vi "Text control 2 v2.7.vi"() -> ()   [LabVIEW 2016]
panel:
  out "Total lines":i32
  out "Line running":i32
  in  "byte count":u32=64
  in  "Serial Settings:Serial End Mode for Reads":u16(ring)=2 items=["None", "LastBit", "TermChar"]
  in  "Timeout (ms)":u32=10000
  in  "Enable Termination\nChar (T)":bool=TRUE
  in  "Termination char\n(0xA = '\\n' = LF)\n(0xD = '\\r' = CR)":u8=13 format="%.0x"
  in  "flow control":u16(ring) items=["None"=0, "XON/XOFF"=1, "RTS/CTS"=2, "DTR/DSR"=4]
  in  "stop bits":u16(ring)=10 items=["1.0"=10, "1.5"=15, "2.0"=20]
  in  "parity":u16(ring) items=["None", "Odd", "Even", "Mark", "Space"]
  in  "data bits":u16=8 min=5 max=8 step=1
  in  "VISA resource name":refnum<visa-resource-name>="COM6"
  in  "baud rate":u32=9600
  out "Serial port output":string
  out "error out":errorcluster
  in  "Units":bool
  out "Elapsed Time":dbl caption="Elapsed Time (s)"
  out "Id max vs time":cluster{"Y data in":dbl[], "X data in":dbl[]}[](graph)
  out "Ig":dbl format="%.2e"
  out "Id":dbl format="%.2e"
  out "Is":dbl format="%.2e"
  out "I vs Vg":cluster{"Y data in":dbl[], "X data in":dbl[]}[](graph)
  in  "Panel Controls 2":T1={"Emergency Stop"=refnum, "TransGraph Max"=1e-05, "Text/Graph (text=false)"=TRUE, "TransGraph Min"=1e-11} {"TransGraph Min" format="%.2e"; "TransGraph Max" format="%.2e"}
  out "Command running:":string="#output s 0 0 0 -0.008 0.008 0.002"
  in  "Standby":T2
  in  "Full Reset":bool
  in  "SMU4":cluster{"on/off":bool, "Voltage":dbl} {"Voltage" min=-100.0 max=100.0 format="%.2f"}
  in  "Source/Drain Range":u8(slide)=6 max=11 scale=0.0..11.0
  in  "Source/Drain\nRange mode":u16(ring) items=["Auto", "Limited", "Fixed"]
  in  "Gate Range":u8(slide)=6 max=11 scale=0.0..11.0
  in  "Gate Range\nmode":u16(ring) items=["Auto", "Limited", "Fixed"]
  in  "Gate":T3={"Gate Start"=0.0, "Gate Stop"=2.0, "Gate Step (linear only)"=1.0, "Gate Compliance"=0.0001, "Gate PComp"=0.0, "Range mode"=0, "Range"=6} {"Range" max=11 scale=0.0..11.0; "Range mode" items=["Auto", "Limited", "Fixed"]; "Gate PComp" format="%^.2e"; "Gate Compliance" format="%^.2e"; "Gate Step (linear only)" format="%^.4e"; "Gate Stop" format="%^.4e"; "Gate Start" format="%^.4e"}
  in  "Drain 2":T4={"Drain Start"=0.0, "Drain Stop"=2.0, "Drain Compliance"=0.0001, "Drain Step"=1.0, "Drain PComp"=0.0, "Range mode"=0, "Range"=6} {"Range" max=11 scale=0.0..11.0; "Range mode" items=["Auto", "Limited", "Fixed"]; "Drain PComp" format="%^.2e"; "Drain Step" format="%^.4e"; "Drain Compliance" format="%^.2e"; "Drain Stop" format="%^.4e"; "Drain Start" format="%^.4e"}
  in  "Timings 2":T5={"integration time"=0, "Short/Long integration time"=0.00064, "hold time (sec)"=0.0, "delay time (sec)"=0.0, "Step Time (0 disables)"=0.0, "sweep method"=0, "Pulse period"=0.005, "Base voltage"=0.0, "Pulse width"=0.0005} {"Pulse width" min=0.0005 max=0.1 step=0.0001 format="%.4f"; "Base voltage" format="%^.4e"; "Pulse period" min=0.005 max=1.0 step=0.0001 format="%.4f"; "sweep method" items=["Continuous", "Pulsed"]; "Step Time (0 disables)" format="%.2f"; "delay time (sec)" format="%.4f"; "hold time (sec)" format="%.4f"; "Short/Long integration time" format="%^.0e"; "integration time" scale=0.0..2.0}
  in  "Panel Controls":T6={"Emergency Stop"=refnum, "TransGraph Max"=1e-05, "Text/Graph (text=false)"=TRUE} {"TransGraph Max" format="%.2e"}
  in  "Interrupt run":bool
  in  "Drain: Compliance":dbl=0.001 format="%.8f"
  in  "Gate: Compliance":dbl=0.001 format="%.8f"
  out "Path":path=path "C:/users/rlp38/09Apr2009LTtesting/test2.txt"
  in  "hold time /s":dbl format="%.2f"
  in  "delay time /s":dbl format="%.2f"
  in  "integration time":u32(slide) max=2 step=1 scale=0.0..2.0
  in  "Integration time (short)":dbl=0.0019 min=8e-05 max=0.0019 step=8e-05 format="%^.0e"
  in  "Integration time (long)":dbl=0.32 min=0.04 max=2.0 step=0.02 format="%.2f"
  in  "Step delay /s":dbl format="%.2f"
  in  "Program":string="#pulsedstressV d 0.03 20 0 0.5 0.0827 5\n#\n#itime s\n#gaterangemode l\n#drainrangemode l\n#pulsed on 0.05 0 0.02\n#transfer d 1 -1 -0.1 -1 -1 0\n#wait-min 1\n#transfer d 1 -1 -0.1 -1 -1 0\n#output d 0 -1 -0.5 0 -1 -0.1\n#transfer d -10 40 1 5 40 35\n#transfer d -10 40 1 5 40 35\n#output d 0 40 20 0 40 1\n#\n#\n#sample 1 0.008 221 6 0.003\n#samplei 400e-6 200 6 0.002 0.1\n#vsu2pulse -10 4\n#\n#stressV 0.016 0.03 2e-4 0.1e-3 11\n#stressI 220e-7 0.08 15\n#transfer s -1 1 0.5 -0.005 0.005 0.005\n#output s 0 0 0 -0.008 0.008 0.002\n"
  # "Serial port settings"
  # "Time"
  # "Sec"
  # "Min"
  # "100 samples is approx 13s with medium integration"
  # "Syntax:\nitime [s|m|l]\ngaterangemode [a|l|f]\ndrainrangemode [a|l|f]\npulsed [on|off] PulsePeriod(sec) PulseBaseVoltage PulseONWidth(sec)\nstandby [on l off]\nwait NumMilliseconds\nwait-min NumMinutes\n# texthere = comment\ntransfer [s|d] VgStart VgStop VgStep VdStart VdStop VdStep\noutput [s|d] VgStart VgStop VgStep VdStart VdStop VdStep\nsample Vg Vd NumSamples Time(s) SampleInterval(s)\nsamplei Idg NumSamples Time(s) SampleInterval(s) VDGcompliance\n# if in doubt use SampleInterval(s) = 0.004\nstressV VG VD IGcompliance IDcompliance Duration(sec)\nstressI IDG VDGcompliance Duration(sec)\nvsu2pulse Bias Duration(s)\npulsedstressV [s|d] VEstop VgON VgOFF Period(s) PulseONwidth(s) Vd\nsample-fpp Vg Vd NumSamples Time\nresample-fpp Vg Vd\ntransfer-fpp [s|d] VgStart VgStop VgStep VdStart VdStop VdStep\noutput-fpp [s|d] VgStart VgStop VgStep VdStart VdStop VdStep\nserial SerialPortCommand"
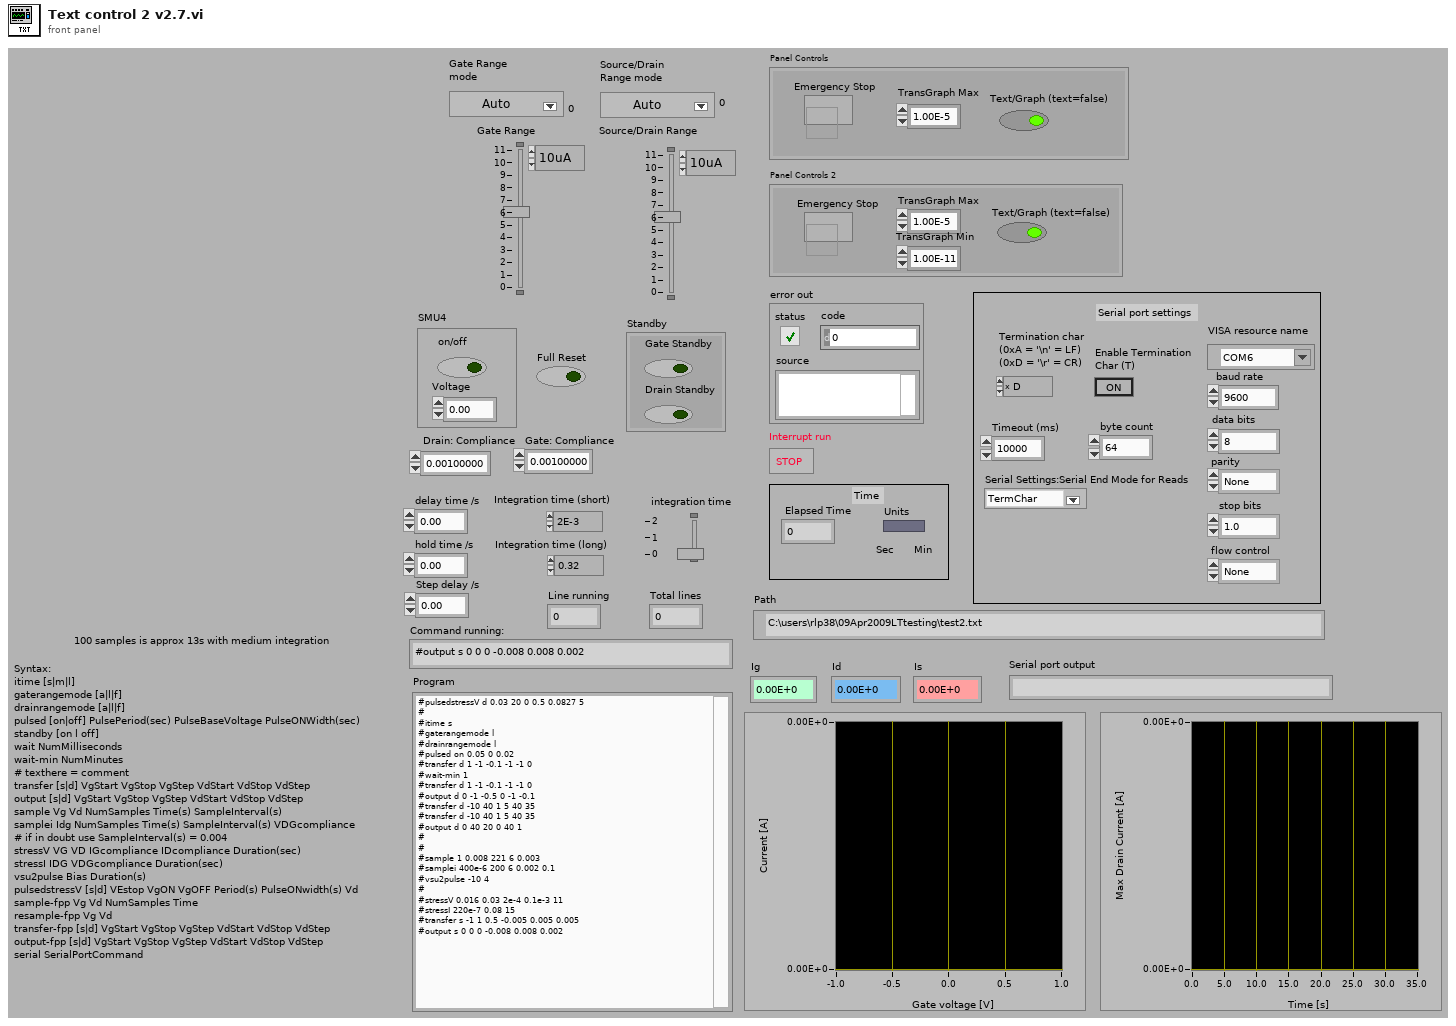
[diagram p1: front panel]
types:
  T1 = cluster{"Emergency Stop":refnum<vi>, "TransGraph Max":dbl, "Text/Graph (text=false)":bool, "TransGraph Min":dbl}
  T2 = cluster{"Gate Standby":bool, "Drain Standby":bool}
  T3 = cluster{"Gate Start":dbl, "Gate Stop":dbl, "Gate Step (linear only)":dbl, "Gate Compliance":dbl, "Gate PComp":dbl, "Range mode":u16, "Range":u8}
  T4 = cluster{"Drain Start":dbl, "Drain Stop":dbl, "Drain Compliance":dbl, "Drain Step":dbl, "Drain PComp":dbl, "Range mode":u16, "Range":u8}
  T5 = cluster{"integration time":u32, "Short/Long integration time":dbl, "hold time (sec)":dbl, "delay time (sec)":dbl, "Step Time (0 disables)":dbl, "sweep method":u16, "Pulse period":dbl, "Base voltage":dbl, "Pulse width":dbl}
  T6 = cluster{"Emergency Stop":refnum<vi>, "TransGraph Max":dbl, "Text/Graph (text=false)":bool}
  T7 = enum16{"open", "replace", "create", "open or create", "replace or create", "replace or create with confirmation"}
  T8 = cluster{"V2 Start":dbl, "V2 Step":dbl, "Number of points":i32}
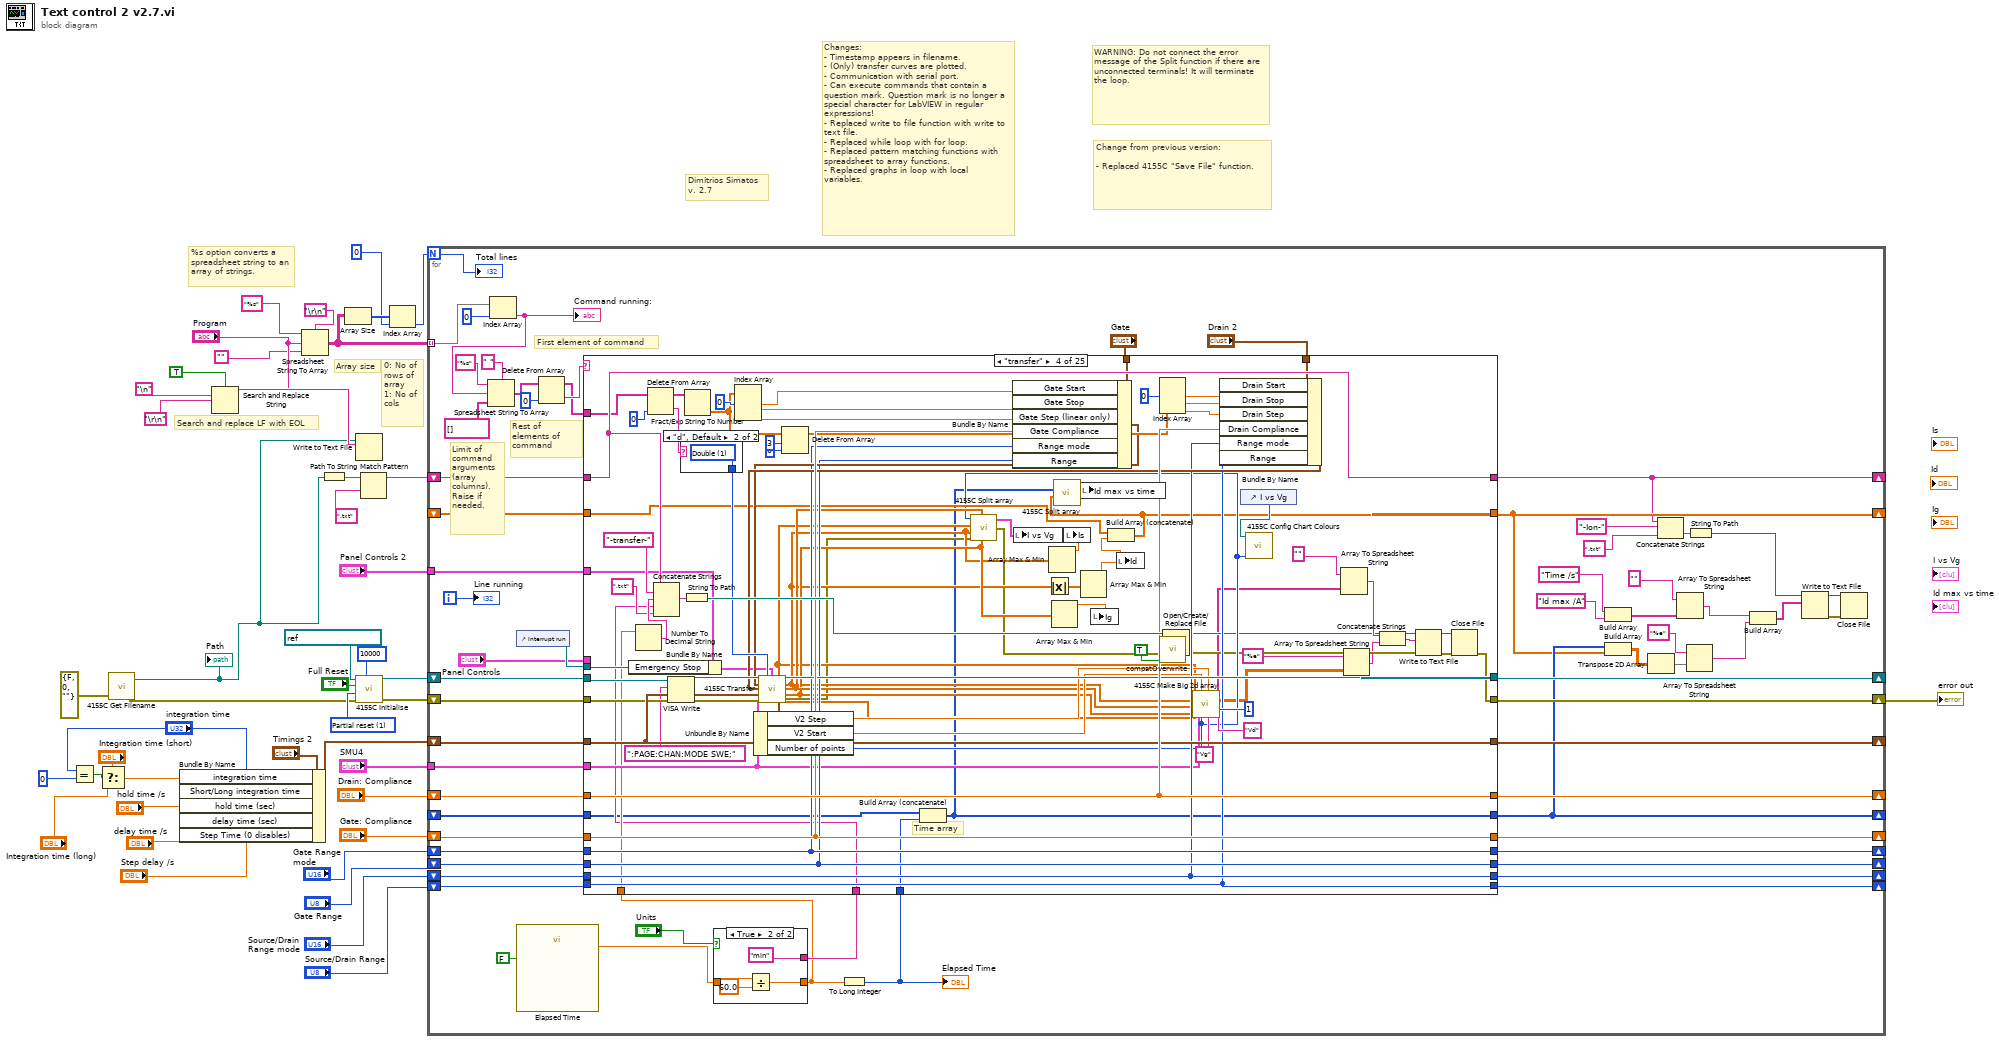
[diagram p0: block diagram]
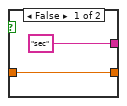
[diagram p2: hidden frame]
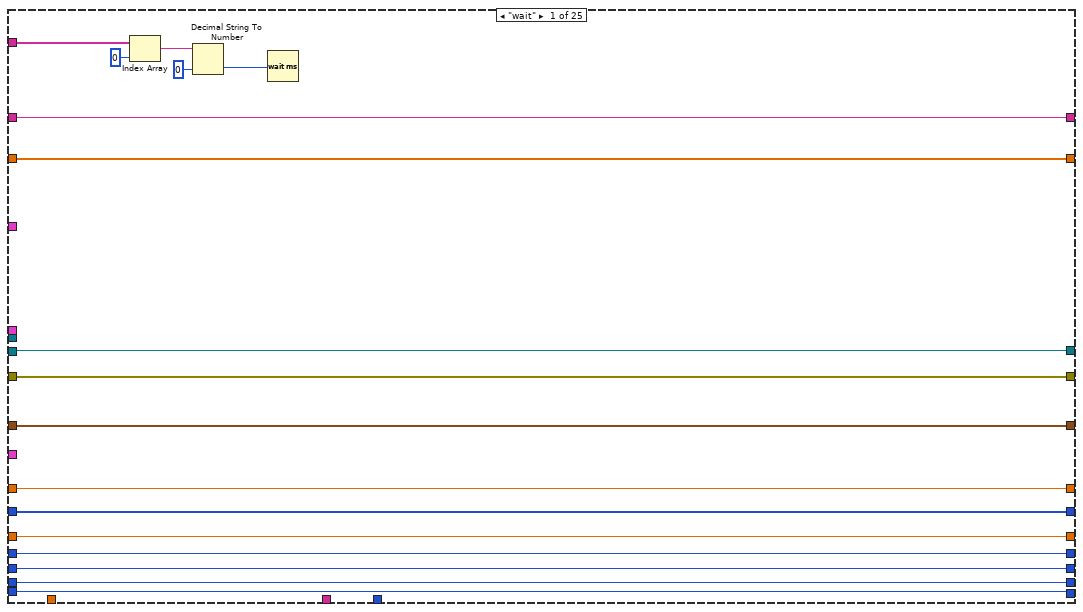
[diagram p3: hidden frame]
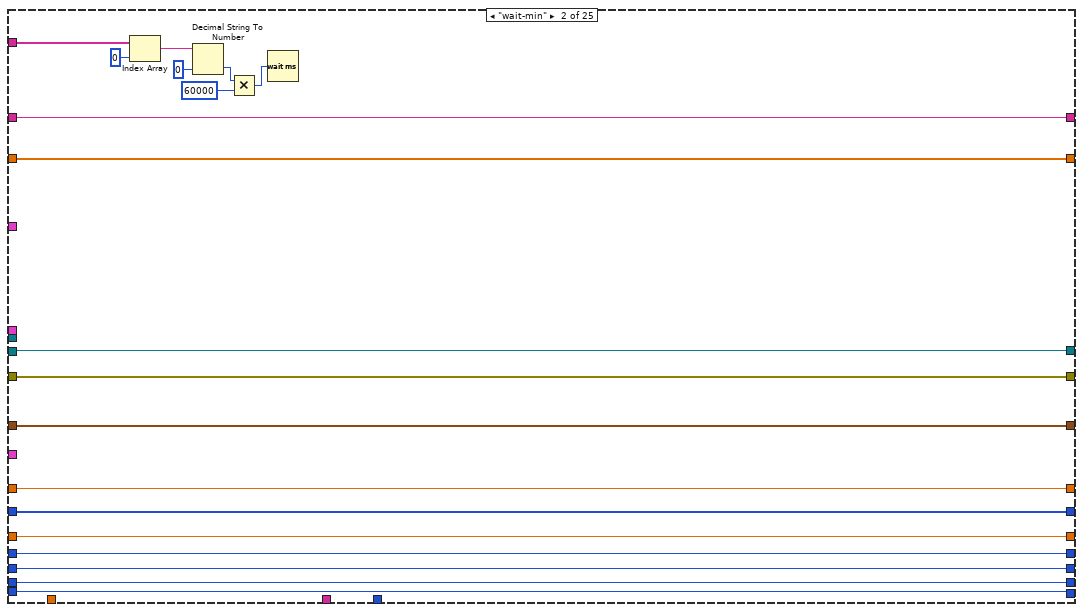
[diagram p4: hidden frame]
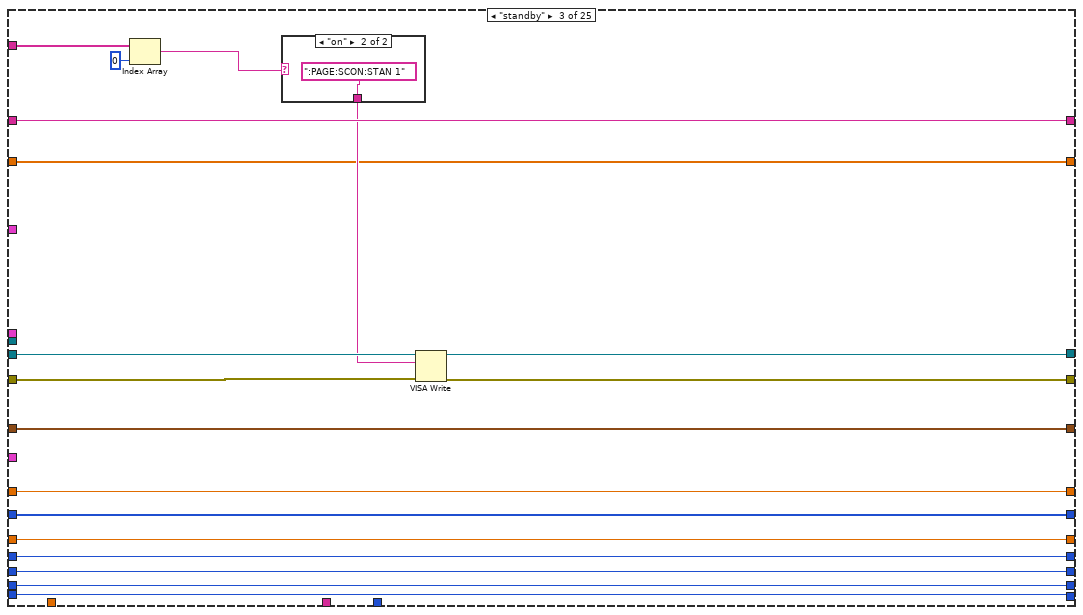
[diagram p5: hidden frame]
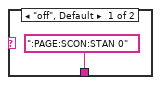
[diagram p6: hidden frame]
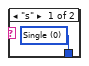
[diagram p7: hidden frame]
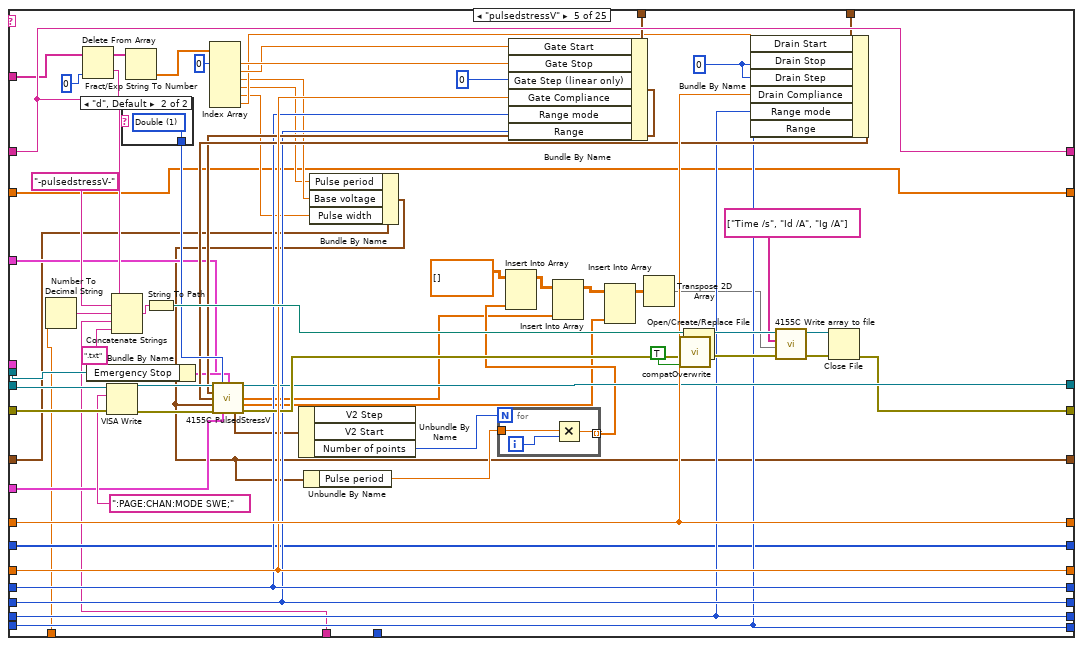
[diagram p8: hidden frame]
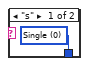
[diagram p9: hidden frame]
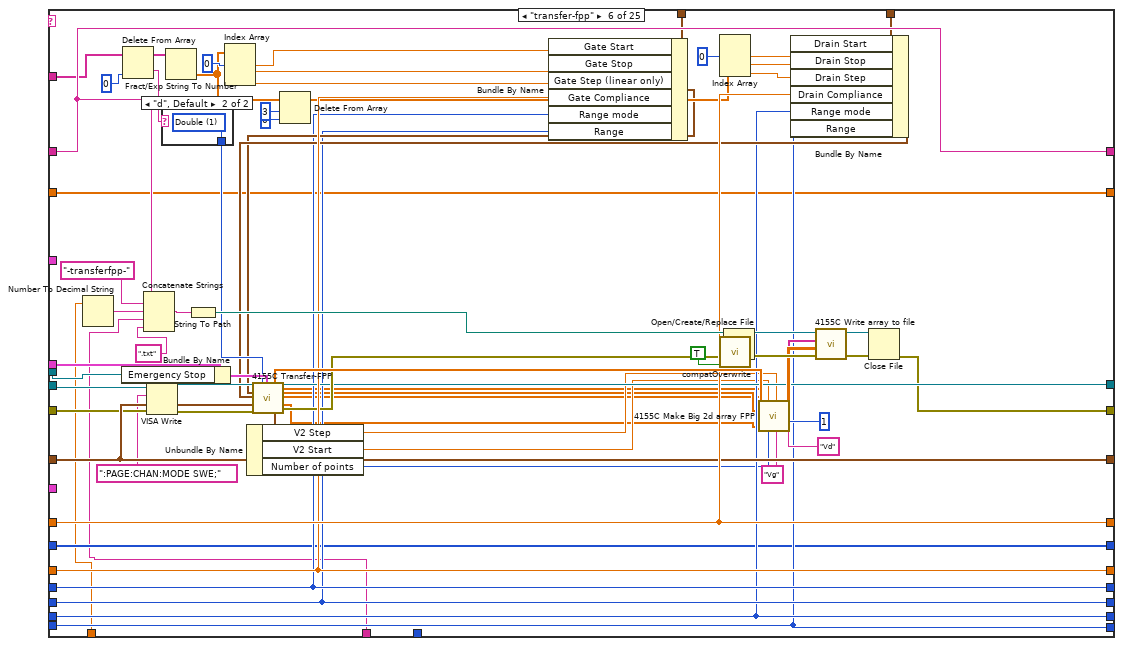
[diagram p10: hidden frame]
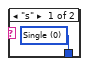
[diagram p11: hidden frame]
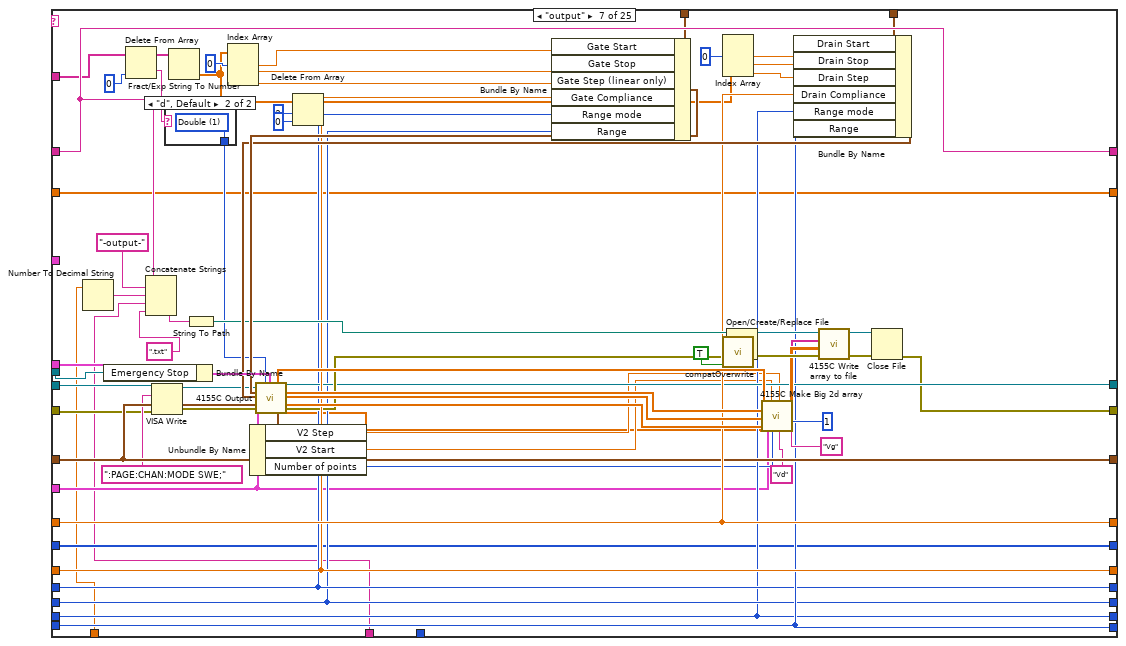
[diagram p12: hidden frame]
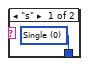
[diagram p13: hidden frame]
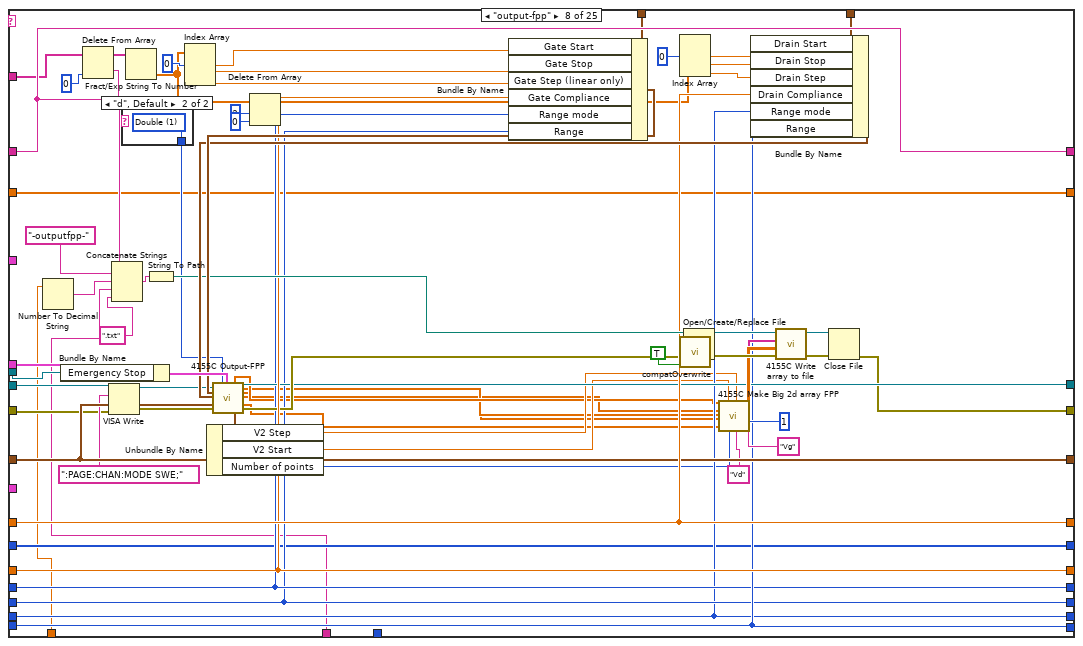
[diagram p14: hidden frame]
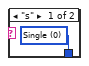
[diagram p15: hidden frame]
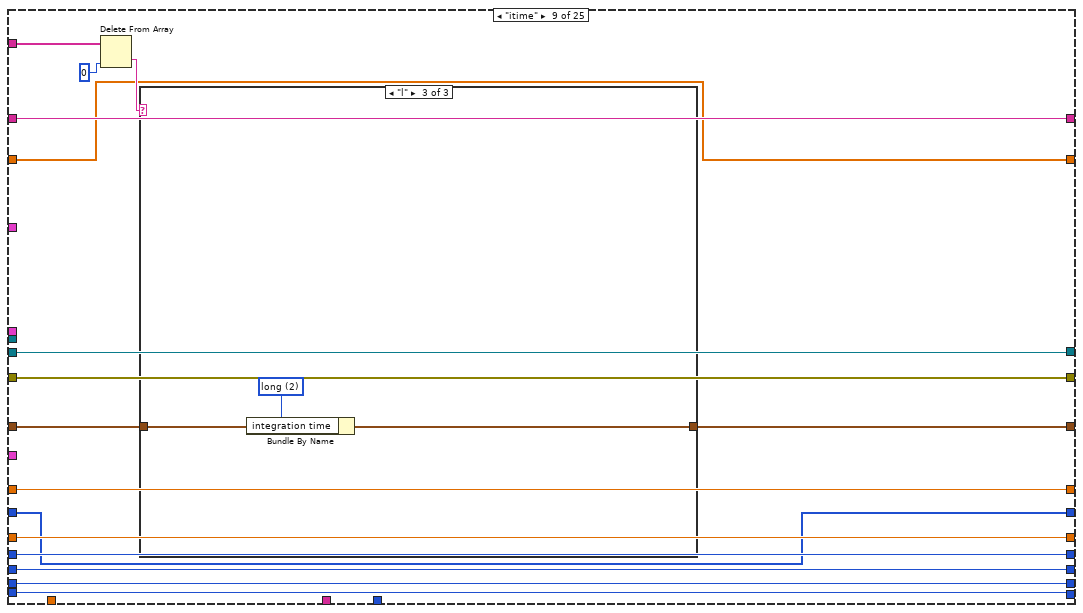
[diagram p16: hidden frame]
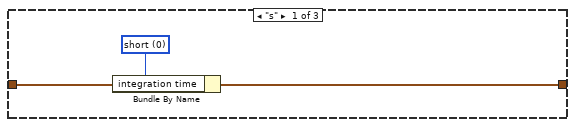
[diagram p17: hidden frame]
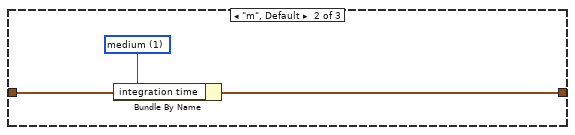
[diagram p18: hidden frame]
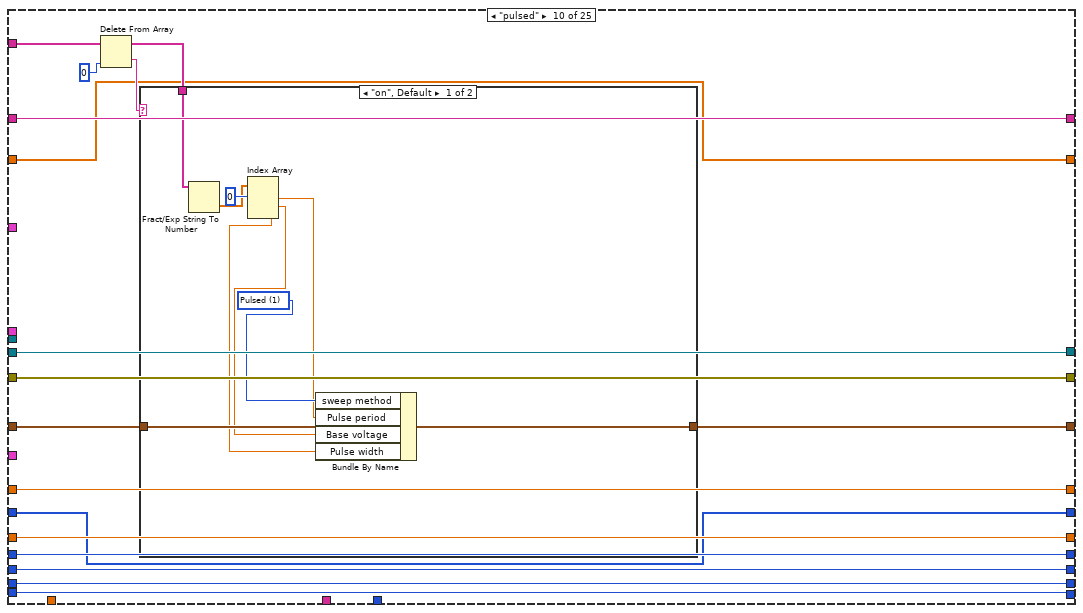
[diagram p19: hidden frame]
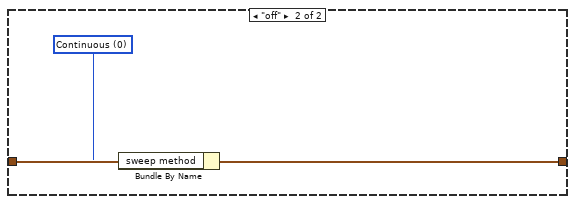
[diagram p20: hidden frame]
diagram:
  w35 = u16 1 items=["Reset All", "Partial reset"] ("Type of reset")
  # "WARNING: Do not connect the error message of the Split function if there are unconnected terminals! It will terminate the loop."
  # "Array size"
  # "%s option converts a spreadsheet string to an array of strings."
  # "0: No of rows of array\n1: No of cols"
  # "Change from previous version:\n\n- Replaced 4155C \"Save File\" function."
  # "Dimitrios Simatos\nv. 2.7"
  # "Changes:\n- Timestamp appears in filename.\n- (Only) transfer curves are plotted.\n- Communication with serial port.\n- Can execute commands that contain a question mark. Question mark is no longer a special character for LabVIEW in regular expressions!\n- Replaced write to file function with write to text file.\n- Replaced while loop with for loop.\n- Replaced pattern matching functions with spreadsheet to array functions.\n- Replaced graphs in loop with local variables."
  # "Search and replace LF with EOL"
  n1 = Equal?(x="integration time", y=u32 0) -> (x = y?=w39:bool)
  n2 = Select(t="Integration time (short)", s=w39, f="Integration time (long)") -> (s? t:f=w43:dbl)
  n3 = call "4155C Get Filename.vi"("error in (no error)"=errorcluster {"status"=FALSE, "code"=0, "source"=""}) -> ("error out"=w30:errorcluster, "path"=w2:path)  [unwired: 2 in, 1 out]
  "Path" <- w2
  n4 = Bundle By Name(cluster="Timings 2", "integration time"="integration time", "Short/Long integration time"=w43, "hold time (sec)"="hold time /s", "delay time (sec)"="delay time /s", "Step Time (0 disables)"="Step delay /s") -> (w27:T5)
  n5 = Search and Replace String(replace all?=TRUE ("replace all? (F)"), input string="Program", search string="\n", replace string="\r\n") -> (result string=w17:string)  [unwired: 4 in, 3 out]
  n6 = Spreadsheet String To Array(delimiter (Tab)="\r\n", format string="%s", spreadsheet string="Program", array type (2D Dbl)="") -> (array=w8:string[][])
  n7 = Path To String(path=w2) -> (string=w5:string)
  n8 = Array Size(array=w8) -> (size(s)=w12:i32[])
  n9 = Write to Text File(file (use dialog)=w2, text=w17) -> ()  [unwired: 2 in, 3 out]
  n10 = call "4155C Initialise.vi"("VISA resource name in"=refnum<visa-resource-name> "GPIB0::14::INSTR", "Reset"="Full Reset", "Type of reset"=w35, "error in (no error)"=w30, "VISA Timeout Value"=u32 10000) -> ("VISA Resource Name out"=w29:refnum<visa-resource-name>, "error out"=w28:errorcluster)
  n11 = Match Pattern(string=w5, regular expression=".txt") -> (before substring=w3:string)  [unwired: 1 in, 3 out]
  n12 = Index Array(array=w12, index=0) -> (element=w10:i32)
  n13 = for {
    N: w10 -> [w72]
    tunnel: "SMU4" -> [w85]
    shift-left: "Source/Drain Range" -> [w90]
    shift-right: [w86] -> _
    shift-left: "Source/Drain\nRange mode" -> [w91]
    shift-right: [w87] -> _
    shift-left: "Gate Range" -> [w92]
    shift-right: [w88] -> _
    shift-left: "Gate Range\nmode" -> [w93]
    shift-right: [w89] -> _
    shift-left: "Gate: Compliance" -> [w103]
    shift-right: [w98] -> _
    shift-left: "Drain: Compliance" -> [w104]
    shift-right: [w99] -> _
    shift-left: w27 -> [w105]
    shift-right: [w100] -> _
    shift-left: w28 -> [w106]
    shift-right: [w101] -> w1
    shift-left: w29 -> [w107]
    shift-right: [w102] -> _
    shift-left: w3 -> [w108]
    shift-right: [w45] -> _
    tunnel: "Panel Controls 2" -> [w84]
    shift-right: [w48] -> _
    shift-left: _ -> [w83]
    shift-right: [w49] -> _
    shift-left: _ -> [w78]
    tunnel: w8 -> [w75] mode=indexing
    i -> [w73]
    # "Limit of command arguments (array columns). Raise if needed."
    # "Rest of elements of command"
    # "First element of command"
    n14 = Index Array(array=w75, index=0 ("line index")) -> (element=w68:string)
    "Command running:" <- w68
    n15 = Spreadsheet String To Array(delimiter (Tab)=" ", format string="%s", spreadsheet string=w68, array type (2D Dbl)=string[] []) -> (array=w65:string[])
    n16 = control-ref of="Interrupt run"() -> (w97:refnum<vi>)
    n17 = call "Elapsed Time"("Auto Reset"=FALSE) -> ("Elapsed Time (s)"=w79:dbl)  [unwired: 11 in, 7 out]
    n18 = Delete From Array(array=w65, index=0) -> (deleted portion=w66:string, array with subset deleted=w64:string[])  [unwired: 1 in]
    n19 = case shown="True" "Units" {
      tunnel: ["sec" "min"] -> w80
      tunnel: [w109 w113] -> w77
      tunnel: w79 -> [w109 w112]
      frame False {
      }
      frame True {
        n20 = Divide(x=w112, y=60.0) -> (x/y=w113:dbl)
      }
    }
    n21 = To Long Integer(number=w77) -> (32bit integer=w76:i32)
    "Elapsed Time" <- w76
    n22 = case shown="\"transfer\"" w66 {
      tunnel: w64 -> [w131 w150 w168 w245 w309 w378 w445 w520 w558 w584 w611 w636 w657 w671 _ _ w775 w836 _ w901 w945 w987 w1057 w1119 w1126]
      tunnel: w108 -> [w126 w146 w166 w252 w316 w386 w453 w528 w547 w573 w603 w629 w651 w664 w683 w725 w753 w818 w849 w888 w932 w975 w1051 w1115 w1128]
      tunnel: w107 -> [w125 w145 w157 w223 w300 w355 w421 w496 w548 w574 w604 w630 w652 w665 w688 w727 w781 w842 w853 w907 w951 w993 w1063 w1073 w1132]
      tunnel: w106 -> [w124 w144 w156 w222 w299 w354 w418 w493 w549 w575 w605 w631 w653 w666 w687 w698 w780 w841 w852 w906 w950 w992 w1062 w1072 w1131]
      tunnel: w105 -> [w123 w143 w165 w248 w275 w382 w449 w524 w557 w583 w602 w628 w650 w663 w686 w722 w744 w810 w858 w881 w925 w968 w1050 w1114 w1133]
      tunnel: w104 -> [w122 w142 w164 w250 w314 w384 w451 w526 w556 w582 w610 w635 w656 w670 w685 w707 w779 w840 w861 w905 w949 w991 w1061 w1123 w1134]
      tunnel: w103 -> [w121 w141 w163 w249 w313 w383 w450 w525 w555 w581 w609 w634 w655 w669 w684 w708 w754 w819 w860 w889 w933 w976 w1052 w1116 w1136]
      tunnel: [w125 w145 w155 w247 w311 w380 w447 w522 w548 w574 w604 w630 w652 w665 w688 w727 w745 w792 w851 w882 w926 w969 w1003 w1075 w1132] -> w102
      tunnel: [w124 w144 w154 w246 w310 w379 w446 w521 w549 w575 w605 w631 w653 w666 w687 w697 w755 w793 w850 w890 w934 w977 w1002 w1074 w1130] -> w101
      tunnel: [w123 w143 w165 w248 w271 w382 w449 w524 w550 w576 w602 w628 w650 w663 w686 w722 w744 w810 w858 w881 w925 w968 w1050 w1114 w1133] -> w100
      tunnel: [w122 w142 w164 w250 w314 w384 w451 w526 w556 w582 w610 w635 w656 w670 w685 w707 w779 w840 w861 w905 w949 w991 w1061 w1123 w1134] -> w99
      tunnel: [w121 w141 w163 w249 w313 w383 w450 w525 w555 w581 w609 w634 w655 w669 w684 w708 w754 w819 w860 w889 w933 w976 w1052 w1116 w1136] -> w98
      tunnel: [w126 w146 w166 w252 w316 w386 w453 w528 w547 w573 w603 w629 w651 w664 w683 w725 w753 w818 w849 w888 w932 w975 w1051 w1115 w1128] -> w45
      tunnel: w97 -> [_ _ _ w255 w320 w391 w461 w532 _ _ _ _ _ _ _ _ w750 w815 _ w887 w931 w974 w1023 w1091 _]
      tunnel: "Gate" -> [_ _ _ w232 w303 w365 w432 w507 _ _ _ _ _ _ _ _ _ _ _ _ _ _ _ _ _]
      tunnel: "Drain 2" -> [_ _ _ w231 w302 w364 w431 w506 _ _ _ _ _ _ _ _ _ _ _ _ _ _ _ _ _]
      tunnel: "Panel Controls" -> [_ _ _ _ _ w363 w430 w505 _ _ _ _ _ _ _ _ _ _ _ _ _ _ _ _ _]
      tunnel: w93 -> [w120 w140 w162 w216 w293 w348 w416 w491 w554 w580 _ w627 w649 w662 w682 w709 w740 w806 w854 w877 w921 w964 w1046 w1110 w1137]
      tunnel: w92 -> [w119 w139 w161 w215 w292 w347 w415 w490 w553 w579 w608 _ w640 w668 w681 w710 w741 w807 w855 w878 w922 w965 w1047 w1111 w1138]
      tunnel: w91 -> [w118 w138 w160 w214 w291 w346 w414 w489 w552 w578 w607 w633 w654 _ w680 w711 w742 w808 w856 w879 w923 w966 w1048 w1112 w1139]
      tunnel: w90 -> [w117 w137 w159 w213 w290 w345 w417 w492 w551 w577 w606 w632 _ w667 w679 w712 w743 w809 w857 w880 w924 w967 w1049 w1113 w1140]
      tunnel: [w120 w140 w162 w216 w293 w348 w416 w491 w554 w580 w601 w627 w649 w662 w682 w709 w740 w806 w854 w877 w921 w964 w1046 w1110 w1137] -> w89
      tunnel: [w119 w139 w161 w215 w292 w347 w415 w490 w553 w579 w608 w619 w640 w668 w681 w710 w741 w807 w855 w878 w922 w965 w1047 w1111 w1138] -> w88
      tunnel: [w118 w138 w160 w214 w291 w346 w414 w489 w552 w578 w607 w633 w654 w661 w680 w711 w742 w808 w856 w879 w923 w966 w1048 w1112 w1139] -> w87
      tunnel: [w117 w137 w159 w213 w290 w345 w417 w492 w551 w577 w606 w632 w641 w667 w679 w712 w743 w809 w857 w880 w924 w967 w1049 w1113 w1140] -> w86
      tunnel: w85 -> [_ _ _ w208 w287 _ w409 _ _ _ _ _ _ _ _ _ _ _ _ _ _ _ _ _ _]
      tunnel: w84 -> [_ _ _ w206 w286 _ _ _ _ _ _ _ _ _ _ _ _ _ _ _ _ _ _ _ _]
      tunnel: [w116 w133 w152 w174 w263 w335 w406 w478 w546 w571 w600 w618 w639 w660 w678 w693 w732 w790 w848 w866 w914 w958 w1000 w1068 w1129] -> w48
      tunnel: w83 -> [w116 w133 w152 w197 w263 w335 w406 w478 w546 w571 w600 w618 w639 w660 w678 w693 w732 w790 w848 w866 w914 w958 w1000 w1068 w1129]
      tunnel: w77 -> [_ _ _ w193 w260 w333 w403 w475 _ _ _ _ _ _ _ w691 w730 w787 _ w863 w911 w955 w997 w1064 _]
      tunnel: w80 -> [_ _ _ w190 w259 w331 w402 w474 _ _ _ _ _ _ _ w689 w728 w786 _ w862 w910 w954 w996 w1065 _]
      tunnel: w76 -> [_ _ _ w175 _ _ _ _ _ _ _ _ _ _ _ _ _ _ _ _ _ _ _ _ _]
      tunnel: [w115 w132 w151 w173 w262 w334 w405 w477 w545 w570 w599 w617 w638 w659 w677 w692 w731 w789 w847 w865 w913 w957 w999 w1067 w1135] -> w49
      tunnel: w78 -> [w115 w132 w151 w189 w262 w334 w405 w477 w545 w570 w599 w617 w638 w659 w677 w692 w731 w789 w847 w865 w913 w957 w999 w1067 w1135]
      frame "wait" {
        n23 = Index Array(array=w131, index=0 ("Index")) -> (element=w129:string)
        n24 = Decimal String To Number(string=w129, default (0L)=u32 0) -> (number=w128:u32)  [unwired: 1 in, 1 out]
        n25 = Wait (ms)(milliseconds to wait=w128) -> ()  [unwired: 1 out]
      }
      frame "wait-min" {
        n26 = Index Array(array=w150, index=0 ("Index")) -> (element=w148:string)
        n27 = Decimal String To Number(string=w148, default (0L)=u32 0) -> (number=w136:u32)  [unwired: 1 in, 1 out]
        n28 = Multiply(x=w136, y=u32 60000) -> (x*y=w135:u32)
        n29 = Wait (ms)(milliseconds to wait=w135) -> ()  [unwired: 1 out]
      }
      frame "standby" {
        n30 = Index Array(array=w168, index=0 ("Index")) -> (element=w158:string)
        n31 = case shown="\"on\"" w158 {
          tunnel: [":PAGE:SCON:STAN 0" ":PAGE:SCON:STAN 1"] -> w153
          frame "off", Default {
          }
          frame "on" {
          }
        }
        n32 = VISA Write(VISA resource name=w157, write buffer=w153, error in (no error)=w156) -> (VISA resource name out=w155:refnum<visa-resource-name>, error out=w154:errorcluster)  [unwired: 1 out]
      }
      frame "transfer" {
        # "Time array"
        n33 = Bundle By Name(cluster=w206, "Emergency Stop"=w255) -> (w207:T1)
        n34 = Number To Decimal String(number=w193) -> (decimal integer string=w192:string)  [unwired: 1 in]
        n35 = Delete From Array(array=w245, index=0 ("Index")) -> (deleted portion=w243:string, array with subset deleted=w242:string[])  [unwired: 1 in]
        n36 = Concatenate Strings(w252, "-transfer-" ("Prefix"), w192, w190, ".txt" ("Suffix")) -> (w254:string)
        n37 = VISA Write(VISA resource name=w223, write buffer=":PAGE:CHAN:MODE SWE;" ("write buffer (\"\")"), error in (no error)=w222) -> (VISA resource name out=w220:refnum<visa-resource-name>, error out=w221:errorcluster)  [unwired: 1 out]
        n38 = case shown="\"d\", Default" w243 {
          tunnel: [w257 w258] -> w241
          frame "s" {
            w257 = u16 0 items=["Single", "Double"] ("sweep mode")
          }
          frame "d", Default {
            w258 = u16 1 items=["Single", "Double"] ("sweep mode")
          }
        }
        n39 = String To Path(string=w254) -> (path=w251:path)
        n40 = Fract/Exp String To Number(string=w242) -> (number=w227:dbl[])  [unwired: 3 in, 1 out]
        n41 = Index Array(array=w227, index #1=0 ("Index")) -> (element #1=w240:dbl, element #2=w239:dbl, element #3=w238:dbl)  [unwired: 2 in]
        n42 = Delete From Array(array=w227, length=3 ("Length"), index=0 ("Index")) -> (array with subset deleted=w225:dbl[])  [unwired: 1 out]
        n43 = Build Array (concatenate)(w189, w175) -> (w173:i32[])
        n44 = Bundle By Name(cluster=w232, "Gate Start"=w240, "Gate Stop"=w239, "Gate Step (linear only)"=w238, "Gate Compliance"=w249, "Range mode"=w216, "Range"=w215) -> (w217:T3)
        n45 = Index Array(array=w225, index #1=0 ("Index")) -> (element #1=w235:dbl, element #2=w234:dbl, element #3=w233:dbl)  [unwired: 2 in]
        n46 = call <vilib>:"compatOverwrite.vi"("overwrite (F)"=TRUE) -> ("overwrite?"=w205:T7)
        n47 = Bundle By Name(cluster=w231, "Drain Start"=w235, "Drain Stop"=w234, "Drain Step"=w233, "Drain Compliance"=w250, "Range mode"=w214, "Range"=w213) -> (w218:T4)
        n48 = call "4155C Transfer.vi"("VISA resource name in"=w220, "Gate"=w217, "Drain"=w218, "Timings"=w248, "error in (no error)"=w221, "SMU4"=w208, "sweep mode"=w241, "Panel Controls"=w207) -> ("VG"=w198:dbl[], "Outparams"=w212:T8, "VISA Resource Name out"=w247:refnum<visa-resource-name>, "IS"=w199:dbl[], "ID"=w204:dbl[], "IG"=w200:dbl[], "error out"=w185:errorcluster, "SMU4"=w209:dbl[])  [unwired: 12 in]
        n49 = Unbundle By Name(w212) -> ("V2 Step"=w211:dbl, "V2 Start"=w210:dbl, "Number of points"=w195:i32)
        n50 = call "4155C Split array.vi"("Number of VAR2 steps"=w195, "Y2 data in"=w204, "X data in"=w198, "Y1 data in"=w199, "Y3 data in"=w200, "error in (no error)"=w185) -> ("Array of clusters"=w188:cluster{"Y data in":dbl[], "X data in":dbl[]}[], "error out"=w186:errorcluster)  [unwired: 1 in]
        n51 = local write "I vs Vg"(w188) -> ()
        n52 = Absolute Value(x=w199) -> (abs(x)=w203:dbl[])
        n53 = Array Max & Min(array=w199) -> (max value=w201:dbl)  [unwired: 3 out]
        n54 = Array Max & Min(array=w200) -> (max value=w202:dbl)  [unwired: 3 out]
        n55 = local write "Is"(w201) -> ()
        n56 = Array Max & Min(array=w203) -> (max value=w196:dbl)  [unwired: 3 out]
        n57 = local write "Ig"(w202) -> ()
        n58 = Build Array (concatenate)(w197, w196) -> (w174:dbl[])
        n59 = call "4155C Split array.vi"("X data in"=w173, "Y1 data in"=w174) -> ("Array of clusters"=w187:cluster{"Y data in":dbl[], "X data in":dbl[]}[])  [unwired: 5 in, 1 out]
        n60 = local write "Id max vs time"(w187) -> ()
        n61 = local write "Id"(w196) -> ()
        n62 = Open/Create/Replace File(file path (use dialog)=w251, error in=w186, operation (0:open)=w205) -> (refnum out=w172:refnum<file>, error out=w182:errorcluster)  [unwired: 3 in, 1 out]
        n63 = call "4155C Make Big 2d array.vi"("1D Var1"=w198, "1d IS"=w199, "1d ID"=w204, "1d IG"=w200, "1d SMU4"=w209, "SMU4"=w208, "VAR2 START"=w210, "Number of VAR2 steps"=w195, "VAR2 STEP"=w211, "VAR1 Name"="Vg", "Decimal places in header"=i8 1, "VAR2 Name"="Vd") -> ("Header array"=w171:string[], "Data array"=w179:dbl[][])  [unwired: 14 in]
        n64 = control-ref of="I vs Vg"() -> (w194:refnum<vi>)
        n65 = call "4155C Config Chart Colours.vi"("Numeric"=w195, "XY Graph 2"=w194) -> ()  [unwired: 6 in]
        n66 = Array To Spreadsheet String(array=w171, 3:"" ("format string")) -> (spreadsheet string=w178:string)  [unwired: 1 in]
        n67 = Array To Spreadsheet String(array=w179, 3:"%e" ("format string")) -> (spreadsheet string=w181:string)  [unwired: 1 in]
        n68 = Concatenate Strings(w178, w181) -> (w180:string)
        n69 = Write to Text File(file (use dialog)=w172, text=w180, error in=w182) -> (refnum out=w184:refnum<file>, error out=w183:errorcluster)  [unwired: 1 in, 1 out]
        n70 = Close File(refnum=w184, error in=w183) -> (error out=w246:errorcluster)  [unwired: 1 out]
      }
      frame "pulsedstressV" {
        w269 = 0
        n71 = Number To Decimal String(number=w260) -> (decimal integer string=w317:string)  [unwired: 1 in]
        n72 = Delete From Array(array=w309, index=0 ("Index")) -> (deleted portion=w307:string, array with subset deleted=w306:string[])  [unwired: 1 in]
        n73 = Bundle By Name(cluster=w286, "Emergency Stop"=w320) -> (w288:T1)
        n74 = VISA Write(VISA resource name=w300, write buffer=":PAGE:CHAN:MODE SWE;" ("write buffer (\"\")"), error in (no error)=w299) -> (VISA resource name out=w297:refnum<visa-resource-name>, error out=w298:errorcluster)  [unwired: 1 out]
        n75 = Concatenate Strings(w316, "-pulsedstressV-" ("Substring"), w317, w259, ".txt" ("Substring")) -> (w319:string)
        n76 = case shown="\"d\", Default" w307 {
          tunnel: [w329 w330] -> w305
          frame "s" {
            w329 = u16 0 items=["Single", "Double"] ("sweep mode")
          }
          frame "d", Default {
            w330 = u16 1 items=["Single", "Double"] ("sweep mode")
          }
        }
        n77 = Fract/Exp String To Number(string=w306) -> (number=w301:dbl[])  [unwired: 3 in, 1 out]
        n78 = String To Path(string=w319) -> (path=w315:path)
        n79 = Index Array(array=w301, index #1=0 ("Index")) -> (element #1=w278:dbl, element #2=w277:dbl, element #3=w274:dbl, element #4=w273:dbl, element #5=w272:dbl, element #6=w276:dbl)  [unwired: 5 in]
        n80 = Bundle By Name(cluster=w275, "Pulse period"=w273, "Base voltage"=w274, "Pulse width"=w272) -> (w271:T5)
        n81 = Unbundle By Name(w271) -> ("Pulse period"=w279:dbl)
        n82 = Bundle By Name(cluster=w303, "Gate Start"=w277, "Gate Stop"=w278, "Gate Step (linear only)"=0, "Gate Compliance"=w313, "Range mode"=w293, "Range"=w292) -> (w294:T3)
        n83 = call <vilib>:"compatOverwrite.vi"("overwrite (F)"=TRUE) -> ("overwrite?"=w264:T7)
        n84 = Bundle By Name(cluster=w302, "Drain Start"=w276, "Drain Stop"=w269, "Drain Step"=w269, "Drain Compliance"=w314, "Range mode"=w291, "Range"=w290) -> (w295:T4)
        n85 = call "4155C PulsedStressV.vi"("VISA resource name in"=w297, "sweep mode"=w305, "Panel Controls"=w288, "Gate"=w294, "Drain"=w295, "Timings"=w271, "error in (no error)"=w298, "SMU4"=w287) -> ("VISA Resource Name out"=w311:refnum<visa-resource-name>, "ID"=w267:dbl[], "IG"=w265:dbl[], "Outparams"=w289:T8, "error out"=w312:errorcluster)  [unwired: 3 in]
        n86 = Unbundle By Name(w289) -> ("Number of points"=w266:i32)  [unwired: 2 out]
        n87 = for {
          N: w266 -> [_]
          tunnel: [w326] -> w268 mode=indexing
          tunnel: w279 -> [w328]
          i -> [w327]
          n88 = Multiply(x=w328, y=w327) -> (x*y=w326:dbl)
        }
        n89 = Insert Into Array(array=dbl[][] [] ("Input Array"), new element=w268) -> (w280:dbl[][])  [unwired: 2 in]
        n90 = Insert Into Array(array=w280, new element=w267) -> (w285:dbl[][])  [unwired: 2 in]
        n91 = Insert Into Array(array=w285, new element=w265) -> (w284:dbl[][])  [unwired: 2 in]
        n92 = Transpose 2D Array(2D array=w284) -> (transposed array=w283:dbl[][])
        n93 = Open/Create/Replace File(file path (use dialog)=w315, error in=w312, operation (0:open)=w264) -> (refnum out=w323:refnum<file>, error out=w324:errorcluster)  [unwired: 3 in, 1 out]
        n94 = call "4155C Write array to file.vi"("Byte Stream File Refnum"=w323, "Header"=string[] ["Time /s", "Id /A", "Ig /A"], "Data Array"=w283, "error in (no error)"=w324) -> ("dup refnum"=w321:refnum<file>, "error out"=w322:errorcluster)  [unwired: 1 in]
        n95 = Close File(refnum=w321, error in=w322) -> (error out=w310:errorcluster)  [unwired: 1 out]
      }
      frame "transfer-fpp" {
        n96 = Number To Decimal String(number=w333) -> (decimal integer string=w387:string)  [unwired: 1 in]
        n97 = Bundle By Name(cluster=w363, "Emergency Stop"=w391) -> (w399:T6)
        n98 = Delete From Array(array=w378, index=0 ("Index")) -> (deleted portion=w376:string, array with subset deleted=w375:string[])  [unwired: 1 in]
        n99 = Concatenate Strings(w386, "-transferfpp-" ("Substring"), w387, w331, ".txt" ("Substring")) -> (w389:string)
        n100 = VISA Write(VISA resource name=w355, write buffer=":PAGE:CHAN:MODE SWE;" ("write buffer (\"\")"), error in (no error)=w354) -> (VISA resource name out=w352:refnum<visa-resource-name>, error out=w353:errorcluster)  [unwired: 1 out]
        n101 = case shown="\"d\", Default" w376 {
          tunnel: [w400 w401] -> w374
          frame "s" {
            w400 = u16 0 items=["Single", "Double"] ("sweep mode")
          }
          frame "d", Default {
            w401 = u16 1 items=["Single", "Double"] ("sweep mode")
          }
        }
        n102 = Fract/Exp String To Number(string=w375) -> (number=w359:dbl[])  [unwired: 3 in, 1 out]
        n103 = String To Path(string=w389) -> (path=w385:path)
        n104 = Index Array(array=w359, index #1=0 ("Index")) -> (element #1=w373:dbl, element #2=w372:dbl, element #3=w371:dbl)  [unwired: 2 in]
        n105 = Delete From Array(array=w359, length=3 ("Length"), index=0 ("Index")) -> (array with subset deleted=w357:dbl[])  [unwired: 1 out]
        n106 = Bundle By Name(cluster=w365, "Gate Start"=w373, "Gate Stop"=w372, "Gate Step (linear only)"=w371, "Gate Compliance"=w383, "Range mode"=w348, "Range"=w347) -> (w349:T3)
        n107 = Index Array(array=w357, index #1=0 ("Index")) -> (element #1=w368:dbl, element #2=w367:dbl, element #3=w366:dbl)  [unwired: 2 in]
        n108 = call <vilib>:"compatOverwrite.vi"("overwrite (F)"=TRUE) -> ("overwrite?"=w336:T7)
        n109 = Bundle By Name(cluster=w364, "Drain Start"=w368, "Drain Stop"=w367, "Drain Step"=w366, "Drain Compliance"=w384, "Range mode"=w346, "Range"=w345) -> (w350:T4)
        n110 = call "4155C Transfer-FPP.vi"("VISA resource name in"=w352, "Gate"=w349, "Drain"=w350, "Timings"=w382, "error in (no error)"=w353, "sweep mode"=w374, "Panel Controls"=w399) -> ("VG"=w390:dbl[], "Outparams"=w344:T8, "VISA Resource Name out"=w380:refnum<visa-resource-name>, "Vprobe2"=w340:dbl[], "ID"=w339:dbl[], "IG"=w338:dbl[], "Vprobe1"=w337:dbl[], "error out"=w381:errorcluster)  [unwired: 13 in]
        n111 = Unbundle By Name(w344) -> ("V2 Step"=w343:dbl, "V2 Start"=w342:dbl, "Number of points"=w341:i32)
        n112 = Open/Create/Replace File(file path (use dialog)=w385, error in=w381, operation (0:open)=w336) -> (refnum out=w396:refnum<file>, error out=w397:errorcluster)  [unwired: 3 in, 1 out]
        n113 = call "4155C Make Big 2d array FPP.vi"("1D Var1"=w390, "1d ID"=w339, "1d Vp2"=w340, "1d IG"=w338, "1d Vp1"=w337, "VAR2 START"=w342, "Number of VAR2 steps"=w341, "VAR2 STEP"=w343, "VAR1 Name"="Vg", "Decimal places in header"=i8 1, "VAR2 Name"="Vd") -> ("Header array"=w392:string[], "Data array"=w393:dbl[][])  [unwired: 15 in]
        n114 = call "4155C Write array to file.vi"("Byte Stream File Refnum"=w396, "Header"=w392, "Data Array"=w393, "error in (no error)"=w397) -> ("dup refnum"=w394:refnum<file>, "error out"=w395:errorcluster)  [unwired: 1 in]
        n115 = Close File(refnum=w394, error in=w395) -> (error out=w379:errorcluster)  [unwired: 1 out]
      }
      frame "output" {
        n116 = Number To Decimal String(number=w403) -> (decimal integer string=w454:string)  [unwired: 1 in]
        n117 = Bundle By Name(cluster=w430, "Emergency Stop"=w461) -> (w471:T6)
        n118 = Delete From Array(array=w445, index=0 ("Index")) -> (deleted portion=w443:string, array with subset deleted=w442:string[])  [unwired: 1 in]
        n119 = Concatenate Strings(w453, "-output-" ("Substring"), w454, w402, ".txt" ("Substring")) -> (w456:string)
        n120 = VISA Write(VISA resource name=w421, write buffer=":PAGE:CHAN:MODE SWE;" ("write buffer (\"\")"), error in (no error)=w418) -> (VISA resource name out=w420:refnum<visa-resource-name>, error out=w419:errorcluster)  [unwired: 1 out]
        n121 = case shown="\"d\", Default" w443 {
          tunnel: [w472 w473] -> w441
          frame "s" {
            w472 = u16 0 items=["Single", "Double"] ("sweep mode")
          }
          frame "d", Default {
            w473 = u16 1 items=["Single", "Double"] ("sweep mode")
          }
        }
        n122 = Fract/Exp String To Number(string=w442) -> (number=w424:dbl[])  [unwired: 3 in, 1 out]
        n123 = String To Path(string=w456) -> (path=w452:path)
        n124 = Index Array(array=w424, index #1=0 ("Index")) -> (element #1=w440:dbl, element #2=w439:dbl, element #3=w438:dbl)  [unwired: 2 in]
        n125 = Delete From Array(array=w424, length=3 ("Length"), index=0 ("Index")) -> (array with subset deleted=w423:dbl[])  [unwired: 1 out]
        n126 = Bundle By Name(cluster=w432, "Gate Start"=w440, "Gate Stop"=w439, "Gate Step (linear only)"=w438, "Gate Compliance"=w450, "Range mode"=w416, "Range"=w415) -> (w470:T3)
        n127 = Index Array(array=w423, index #1=0 ("Index")) -> (element #1=w435:dbl, element #2=w434:dbl, element #3=w433:dbl)  [unwired: 2 in]
        n128 = call <vilib>:"compatOverwrite.vi"("overwrite (F)"=TRUE) -> ("overwrite?"=w407:T7)
        n129 = Bundle By Name(cluster=w431, "Drain Start"=w435, "Drain Stop"=w434, "Drain Step"=w433, "Drain Compliance"=w451, "Range mode"=w414, "Range"=w417) -> (w469:T4)
        n130 = call "4155C Output.vi"("VISA resource name in"=w420, "Gate"=w470, "Drain"=w469, "Timings"=w449, "error in (no error)"=w419, "SMU4"=w409, "sweep mode"=w441, "Panel controls"=w471) -> ("VD"=w457:dbl[], "Outparams"=w412:T8, "VISA Resource Name out"=w447:refnum<visa-resource-name>, "IS"=w460:dbl[], "ID"=w459:dbl[], "IG"=w458:dbl[], "error out"=w448:errorcluster, "SMU4"=w408:dbl[])  [unwired: 12 in]
        n131 = Unbundle By Name(w412) -> ("V2 Step"=w413:dbl, "V2 Start"=w411:dbl, "Number of points"=w410:i32)
        n132 = Open/Create/Replace File(file path (use dialog)=w452, error in=w448, operation (0:open)=w407) -> (refnum out=w466:refnum<file>, error out=w467:errorcluster)  [unwired: 3 in, 1 out]
        n133 = call "4155C Make Big 2d array.vi"("1D Var1"=w457, "1d IS"=w460, "1d ID"=w459, "1d IG"=w458, "1d SMU4"=w408, "SMU4"=w409, "VAR2 START"=w411, "Number of VAR2 steps"=w410, "VAR2 STEP"=w413, "VAR1 Name"="Vd", "Decimal places in header"=i8 1, "VAR2 Name"="Vg") -> ("Header array"=w462:string[], "Data array"=w463:dbl[][])  [unwired: 14 in]
        n134 = call "4155C Write array to file.vi"("Byte Stream File Refnum"=w466, "Header"=w462, "Data Array"=w463, "error in (no error)"=w467) -> ("dup refnum"=w464:refnum<file>, "error out"=w465:errorcluster)  [unwired: 1 in]
        n135 = Close File(refnum=w464, error in=w465) -> (error out=w446:errorcluster)  [unwired: 1 out]
      }
      frame "output-fpp" {
        n136 = Number To Decimal String(number=w475) -> (decimal integer string=w529:string)  [unwired: 1 in]
        n137 = Bundle By Name(cluster=w505, "Emergency Stop"=w532) -> (w542:T6)
        n138 = Delete From Array(array=w520, index=0 ("Index")) -> (deleted portion=w518:string, array with subset deleted=w517:string[])  [unwired: 1 in]
        n139 = VISA Write(VISA resource name=w496, write buffer=":PAGE:CHAN:MODE SWE;" ("write buffer (\"\")"), error in (no error)=w493) -> (VISA resource name out=w495:refnum<visa-resource-name>, error out=w494:errorcluster)  [unwired: 1 out]
        n140 = Concatenate Strings(w528, "-outputfpp-" ("Substring"), w529, w474, ".txt" ("Substring")) -> (w531:string)
        n141 = case shown="\"d\", Default" w518 {
          tunnel: [w543 w544] -> w516
          frame "s" {
            w543 = u16 0 items=["Single", "Double"] ("sweep mode")
          }
          frame "d", Default {
            w544 = u16 1 items=["Single", "Double"] ("sweep mode")
          }
        }
        n142 = Fract/Exp String To Number(string=w517) -> (number=w499:dbl[])  [unwired: 3 in, 1 out]
        n143 = String To Path(string=w531) -> (path=w527:path)
        n144 = Index Array(array=w499, index #1=0 ("Index")) -> (element #1=w515:dbl, element #2=w514:dbl, element #3=w513:dbl)  [unwired: 2 in]
        n145 = Delete From Array(array=w499, length=3 ("Length"), index=0 ("Index")) -> (array with subset deleted=w498:dbl[])  [unwired: 1 out]
        n146 = Bundle By Name(cluster=w507, "Gate Start"=w515, "Gate Stop"=w514, "Gate Step (linear only)"=w513, "Gate Compliance"=w525, "Range mode"=w491, "Range"=w490) -> (w541:T3)
        n147 = Index Array(array=w498, index #1=0 ("Index")) -> (element #1=w510:dbl, element #2=w509:dbl, element #3=w508:dbl)  [unwired: 2 in]
        n148 = call <vilib>:"compatOverwrite.vi"("overwrite (F)"=TRUE) -> ("overwrite?"=w479:T7)
        n149 = Bundle By Name(cluster=w506, "Drain Start"=w510, "Drain Stop"=w509, "Drain Step"=w508, "Drain Compliance"=w526, "Range mode"=w489, "Range"=w492) -> (w540:T4)
        n150 = call "4155C Output-FPP.vi"("VISA resource name in"=w495, "Gate"=w541, "Drain"=w540, "Timings"=w524, "error in (no error)"=w494, "sweep mode"=w516, "Panel controls"=w542) -> ("VD"=w484:dbl[], "Outparams"=w487:T8, "VISA Resource Name out"=w522:refnum<visa-resource-name>, "Vprobe2"=w483:dbl[], "ID"=w482:dbl[], "IG"=w481:dbl[], "Vprobe1"=w480:dbl[], "error out"=w523:errorcluster)  [unwired: 13 in]
        n151 = Unbundle By Name(w487) -> ("V2 Step"=w488:dbl, "V2 Start"=w486:dbl, "Number of points"=w485:i32)
        n152 = Open/Create/Replace File(file path (use dialog)=w527, error in=w523, operation (0:open)=w479) -> (refnum out=w537:refnum<file>, error out=w538:errorcluster)  [unwired: 3 in, 1 out]
        n153 = call "4155C Make Big 2d array FPP.vi"("1D Var1"=w484, "1d ID"=w482, "1d Vp2"=w483, "1d IG"=w481, "1d Vp1"=w480, "VAR2 START"=w486, "Number of VAR2 steps"=w485, "VAR2 STEP"=w488, "VAR1 Name"="Vd", "Decimal places in header"=i8 1, "VAR2 Name"="Vg") -> ("Header array"=w533:string[], "Data array"=w534:dbl[][])  [unwired: 15 in]
        n154 = call "4155C Write array to file.vi"("Byte Stream File Refnum"=w537, "Header"=w533, "Data Array"=w534, "error in (no error)"=w538) -> ("dup refnum"=w535:refnum<file>, "error out"=w536:errorcluster)  [unwired: 1 in]
        n155 = Close File(refnum=w535, error in=w536) -> (error out=w521:errorcluster)  [unwired: 1 out]
      }
      frame "itime" {
        n156 = Delete From Array(array=w558, index=0 ("Index")) -> (deleted portion=w559:string)  [unwired: 1 in, 1 out]
        n157 = case shown="\"l\"" w559 {
          tunnel: w557 -> [w563 w565 w568]
          tunnel: [w562 w564 w567] -> w550
          frame "s" {
            w561 = u32 0 items=["short  ", "medium  ", "long  "] ("integration time 2")
            n158 = Bundle By Name(cluster=w563, "integration time"=w561) -> (w562:T5)
          }
          frame "m", Default {
            w566 = u32 1 items=["short  ", "medium  ", "long  "] ("integration time 2")
            n159 = Bundle By Name(cluster=w565, "integration time"=w566) -> (w564:T5)
          }
          frame "l" {
            w569 = u32 2 items=["short  ", "medium  ", "long  "] ("integration time 2")
            n160 = Bundle By Name(cluster=w568, "integration time"=w569) -> (w567:T5)
          }
        }
      }
      frame "pulsed" {
        n161 = Delete From Array(array=w584, index=0 ("Index")) -> (deleted portion=w585:string, array with subset deleted=w572:string[])  [unwired: 1 in]
        n162 = case shown="\"on\", Default" w585 {
          tunnel: w583 -> [w595 w598]
          tunnel: [w594 w597] -> w576
          tunnel: w572 -> [w592 _]
          frame "on", Default {
            w593 = u16 1 items=["Continuous", "Pulsed"] ("sweep method")
            n163 = Fract/Exp String To Number(string=w592) -> (number=w590:dbl[])  [unwired: 3 in, 1 out]
            n164 = Index Array(array=w590, index #1=0 ("Index")) -> (element #1=w589:dbl, element #2=w588:dbl, element #3=w587:dbl)  [unwired: 2 in]
            n165 = Bundle By Name(cluster=w595, "sweep method"=w593, "Pulse period"=w589, "Base voltage"=w588, "Pulse width"=w587) -> (w594:T5)
          }
          frame "off" {
            w596 = u16 0 items=["Continuous", "Pulsed"] ("sweep method")
            n166 = Bundle By Name(cluster=w598, "sweep method"=w596) -> (w597:T5)
          }
        }
      }
      frame "gaterangemode" {
        n167 = Delete From Array(array=w611, index=0 ("Index")) -> (deleted portion=w612:string)  [unwired: 1 in, 1 out]
        n168 = case shown="\"f\"" w612 {
          tunnel: [w614 w615 w616] -> w601
          frame "a", Default {
            w614 = u16 0 items=["Auto", "Limited", "Fixed"] ("Gate Range\nmode 2")
          }
          frame "f" {
            w615 = u16 2 items=["Auto", "Limited", "Fixed"] ("Gate Range\nmode 2")
          }
          frame "l" {
            w616 = u16 1 items=["Auto", "Limited", "Fixed"] ("Gate Range\nmode 2")
          }
        }
      }
      frame "gaterange" {
        (unwired) u8 11 items=["10fA  ", "100fA  ", "1nA  ", "10nA", "100nA", "1uA", "10uA", "100uA", "1mA", "10mA", "100mA", "1A"] ("Gate Range 2")
        n169 = Delete From Array(array=w636, index=0 ("Index")) -> (deleted portion=w626:string)  [unwired: 1 in, 1 out]
        n170 = Scan Value(string=w626, format string="") -> (value=w624:dbl)  [unwired: 1 in, 1 out]
        n171 = Logarithm Base 10(1:w624) -> (0:w623:dbl)
        n172 = Round To Nearest(number=w623) -> (nearest integer value=w622:dbl)
        n173 = Add(x=w622, y=11.0) -> (x+y=w620:dbl)
        n174 = To Unsigned Byte Integer(number=w620) -> (unsigned 8bit integer=w619:u8)
      }
      frame "drainrange" {
        (unwired) u8 11 items=["10fA  ", "100fA  ", "1nA  ", "10nA", "100nA", "1uA", "10uA", "100uA", "1mA", "10mA", "100mA", "1A"] ("Gate Range 2")
        n175 = Delete From Array(array=w657, index=0 ("Index")) -> (deleted portion=w648:string)  [unwired: 1 in, 1 out]
        n176 = Scan Value(string=w648, format string="") -> (value=w646:dbl)  [unwired: 1 in, 1 out]
        n177 = Logarithm Base 10(1:w646) -> (0:w645:dbl)
        n178 = Round To Nearest(number=w645) -> (nearest integer value=w644:dbl)
        n179 = Add(x=w644, y=11.0) -> (x+y=w642:dbl)
        n180 = To Unsigned Byte Integer(number=w642) -> (unsigned 8bit integer=w641:u8)
      }
      frame "drainrangemode" {
        n181 = Delete From Array(array=w671, index=0 ("Index")) -> (deleted portion=w672:string)  [unwired: 1 in, 1 out]
        n182 = case shown="\"f\"" w672 {
          tunnel: [w674 w675 w676] -> w661
          frame "a", Default {
            w674 = u16 0 items=["Auto", "Limited", "Fixed"] ("Gate Range\nmode 2")
          }
          frame "f" {
            w675 = u16 2 items=["Auto", "Limited", "Fixed"] ("Gate Range\nmode 2")
          }
          frame "l" {
            w676 = u16 1 items=["Auto", "Limited", "Fixed"] ("Gate Range\nmode 2")
          }
        }
      }
      frame "Error", Default {
      }
      frame "logfile" {
        n183 = Number To Decimal String(number=w691) -> (decimal integer string=w726:string)  [unwired: 1 in]
        n184 = Concatenate Strings(w725, "logfile" ("Substring"), w726, w689, ".txt" ("Substring")) -> (w723:string)
        n185 = String To Path(string=w723) -> (path=w696:path)
        n186 = Unbundle(w722) -> ("integration time"=w721:u32, "Short/Long integration time"=w720:dbl, "hold time (sec)"=w719:dbl, "delay time (sec)"=w718:dbl, "Step Time (0 disables)"=w717:dbl, "sweep method"=w716:u16, "Pulse period"=w715:dbl, "Base voltage"=w714:dbl, "Pulse width"=w713:dbl)
        n187 = Build Array(w721, w720, w719, w718, w717, w716, w715, w714, w713, w707, w708, w709, w710, w711, w712) -> (w700:dbl[])
        n188 = Insert Into Array(array=dbl[][] [] ("Input Array"), new element=w700) -> (w699:dbl[][])  [unwired: 2 in]
        n189 = call <vilib>:"compatOverwrite.vi"("overwrite (F)"=TRUE) -> ("overwrite?"=w694:T7)
        n190 = Open/Create/Replace File(file path (use dialog)=w696, error in=w698, operation (0:open)=w694) -> (refnum out=w704:refnum<file>, error out=w703:errorcluster)  [unwired: 3 in, 1 out]
        n191 = call "4155C Write array to file.vi"("Byte Stream File Refnum"=w704, "Header"=string[] ["Int Time", "Short/Long Itime", "Hold time", "Delay time", "Step time", "Sweep method", "Pulse period", "Base Voltage", "Pulse width", "Drain compliance", "Gate compliance", "Gate range mode", "Gate range", "S/D range mode", "S/D range"], "Data Array"=w699, "error in (no error)"=w703) -> ("dup refnum"=w706:refnum<file>, "error out"=w705:errorcluster)  [unwired: 1 in]
        n192 = Close File(refnum=w706, error in=w705) -> (error out=w697:errorcluster)  [unwired: 1 out]
      }
      frame "sample" {
        n193 = Number To Decimal String(number=w730) -> (decimal integer string=w778:string)  [unwired: 1 in]
        n194 = Fract/Exp String To Number(string=w775) -> (number=w736:dbl[])  [unwired: 3 in, 1 out]
        n195 = Concatenate Strings(w753, "-sample-" ("Substring"), w778, w728, ".txt" ("Substring")) -> (w776:string)
        n196 = String To Path(string=w776) -> (path=w757:path)
        n197 = Index Array(array=w736, index=0 ("Index")) -> (element=w773:dbl)
        n198 = Index Array(array=w736, index=2 ("Index")) -> (element=w769:dbl)
        n199 = Index Array(array=w736, index=3 ("Index")) -> (element=w738:dbl)
        n200 = Index Array(array=w736, index=4 ("Index")) -> (element=w735:dbl)
        n201 = call "4155C Config Sampling Measurements.vi"("Sampling interval"=w735, "Sample time"=w738, "Display on/off"=TRUE, "Timings"=w744, "Num Points"=w769, "error in (no error)"=w780, "Drain Compliance"=w779, "Gate Compliance"=w754, "VISA session"=w781) -> ("error out"=w782:errorcluster, "dup VISA resource name"=w783:refnum<visa-resource-name>)  [unwired: 1 in]
        n202 = Index Array(array=w736, index=1 ("Index")) -> (element=w770:dbl)
        n203 = call "4155C Take Sample.vi"("Emergency Stop"=w750, "error in (no error)"=w782, "Vd"=w770, "Vg"=w773, "VISA resource name in"=w783) -> ("error out"=w748:errorcluster, "Id"=w785:dbl[], "Ig"=w759:dbl[], "VISA Resource Name out"=w746:refnum<visa-resource-name>, "Is"=w784:dbl[], "Time"=w763:dbl[])  [unwired: 1 in]
        n204 = Insert Into Array(array=dbl[][] [] ("Input Array"), new element=w763) -> (w762:dbl[][])  [unwired: 2 in]
        n205 = Insert Into Array(array=w762, new element=w759) -> (w761:dbl[][])  [unwired: 2 in]
        n206 = Insert Into Array(array=w761, new element=w785) -> (w760:dbl[][])  [unwired: 2 in]
        n207 = VISA Write(VISA resource name=w746, write buffer=":DISP ON" ("write buffer (\"\")"), error in (no error)=w748) -> (VISA resource name out=w745:refnum<visa-resource-name>, error out=w747:errorcluster)  [unwired: 1 out]
        n208 = Insert Into Array(array=w760, new element=w784) -> (w752:dbl[][])  [unwired: 2 in]
        n209 = Transpose 2D Array(2D array=w752) -> (transposed array=w751:dbl[][])
        n210 = call <vilib>:"compatOverwrite.vi"("overwrite (F)"=TRUE) -> ("overwrite?"=w733:T7)
        n211 = Open/Create/Replace File(file path (use dialog)=w757, error in=w747, operation (0:open)=w733) -> (refnum out=w766:refnum<file>, error out=w765:errorcluster)  [unwired: 3 in, 1 out]
        n212 = call "4155C Write array to file.vi"("Byte Stream File Refnum"=w766, "Header"=string[] ["Time /s", "Ig /A", "Id /A", "Is /A"], "Data Array"=w751, "error in (no error)"=w765) -> ("dup refnum"=w768:refnum<file>, "error out"=w767:errorcluster)  [unwired: 1 in]
        n213 = Close File(refnum=w768, error in=w767) -> (error out=w755:errorcluster)  [unwired: 1 out]
      }
      frame "samplei" {
        n214 = Number To Decimal String(number=w787) -> (decimal integer string=w839:string)  [unwired: 1 in]
        n215 = Fract/Exp String To Number(string=w836) -> (number=w803:dbl[])  [unwired: 3 in, 1 out]
        n216 = Concatenate Strings(w818, "-samplei-" ("Substring"), w839, w786, ".txt" ("Substring")) -> (w837:string)
        n217 = String To Path(string=w837) -> (path=w821:path)
        n218 = Index Array(array=w803, index=4 ("Index")) -> (element=w797:dbl)
        n219 = Index Array(array=w803, index=3 ("Index")) -> (element=w798:dbl)
        n220 = Index Array(array=w803, index=1 ("Index")) -> (element=w800:dbl)
        n221 = Index Array(array=w803, index=0 ("Index")) -> (element=w801:dbl)
        n222 = Index Array(array=w803, index=2 ("Index")) -> (element=w799:dbl)
        n223 = call "4155C Config SamplingI Measurements.vi"("Sample time"=w799, "Display on/off"=TRUE, "Timings"=w810, "Num Points"=w800, "error in (no error)"=w841, "Sampling interval"=w798, "VISA session"=w842) -> ("error out"=w843:errorcluster, "dup VISA resource name"=w844:refnum<visa-resource-name>)  [unwired: 3 in]
        n224 = call "4155C Take SampleI.vi"("Emergency Stop"=w815, "error in (no error)"=w843, "Idg 2"=w801, "Vdg compliance 2"=w797, "VISA resource name in"=w844) -> ("error out"=w813:errorcluster, "Idg"=w846:dbl[], "Vdg"=w823:dbl[], "VISA Resource Name out"=w811:refnum<visa-resource-name>, "Is"=w845:dbl[], "Time"=w827:dbl[])  [unwired: 1 in]
        n225 = Insert Into Array(array=dbl[][] [] ("Input Array"), new element=w827) -> (w826:dbl[][])  [unwired: 2 in]
        n226 = Insert Into Array(array=w826, new element=w823) -> (w825:dbl[][])  [unwired: 2 in]
        n227 = Insert Into Array(array=w825, new element=w846) -> (w824:dbl[][])  [unwired: 2 in]
        n228 = VISA Write(VISA resource name=w811, write buffer=":DISP ON" ("write buffer (\"\")"), error in (no error)=w813) -> (VISA resource name out=w796:refnum<visa-resource-name>, error out=w812:errorcluster)  [unwired: 1 out]
        n229 = Insert Into Array(array=w824, new element=w845) -> (w817:dbl[][])  [unwired: 2 in]
        n230 = Transpose 2D Array(2D array=w817) -> (transposed array=w816:dbl[][])
        n231 = call <vilib>:"compatOverwrite.vi"("overwrite (F)"=TRUE) -> ("overwrite?"=w791:T7)
        n232 = Open/Create/Replace File(file path (use dialog)=w821, error in=w812, operation (0:open)=w791) -> (refnum out=w830:refnum<file>, error out=w829:errorcluster)  [unwired: 3 in, 1 out]
        n233 = call "4155C Write array to file.vi"("Byte Stream File Refnum"=w830, "Header"=string[] ["Time /s", "Vdg /V", "Idg /A", "Is /A"], "Data Array"=w816, "error in (no error)"=w829) -> ("dup refnum"=w832:refnum<file>, "error out"=w831:errorcluster)  [unwired: 1 in]
        n234 = Close File(refnum=w832, error in=w831) -> (error out=w794:errorcluster)  [unwired: 1 out]
        n235 = VISA Write(VISA resource name=w796, write buffer=";:PAGE:SCON:STAN OFF;:PAGE:CHAN:VSU2:DIS;" ("write buffer (\"\")"), error in (no error)=w794) -> (VISA resource name out=w792:refnum<visa-resource-name>, error out=w793:errorcluster)  [unwired: 1 out]
      }
      frame "#" {
        n236 = VISA Write(VISA resource name=w853, write buffer=":DISP ON" ("write buffer (\"\")"), error in (no error)=w852) -> (VISA resource name out=w851:refnum<visa-resource-name>, error out=w850:errorcluster)  [unwired: 1 out]
      }
      frame "stressV" {
        n237 = Number To Decimal String(number=w863) -> (decimal integer string=w904:string)  [unwired: 1 in]
        n238 = Fract/Exp String To Number(string=w901) -> (number=w874:dbl[])  [unwired: 3 in, 1 out]
        n239 = Concatenate Strings(w888, "-stressV-" ("Substring"), w904, w862, ".txt" ("Substring")) -> (w902:string)
        n240 = String To Path(string=w902) -> (path=w892:path)
        n241 = Index Array(array=w874, index=3 ("Index")) -> (element=w871:dbl)
        n242 = Index Array(array=w874, index=1 ("Index")) -> (element=w869:dbl)
        n243 = Index Array(array=w874, index=0 ("Index")) -> (element=w868:dbl)
        n244 = Index Array(array=w874, index=4 ("Index")) -> (element=w873:dbl)
        n245 = Index Array(array=w874, index=2 ("Index")) -> (element=w870:dbl)
        n246 = call "4155C Config V Stress.vi"("VISA session"=w907, "ID compliance"=w871, "VD"=w869, "VG"=w868, "IG compliance"=w870, "error in (no error)"=w906, "Display on/off"=TRUE) -> ("dup VISA resource name"=w909:refnum<visa-resource-name>, "error out"=w908:errorcluster)
        n247 = call "4155C Apply Stress.vi"("error in (no error)"=w908, "Duration"=w873, "Emergency Stop"=w887, "VISA resource name in"=w909) -> ("error out"=w885:errorcluster, "VISA Resource Name out"=w883:refnum<visa-resource-name>)
        n248 = VISA Write(VISA resource name=w883, write buffer=":DISP ON" ("write buffer (\"\")"), error in (no error)=w885) -> (VISA resource name out=w882:refnum<visa-resource-name>, error out=w884:errorcluster)  [unwired: 1 out]
        n249 = call <vilib>:"compatOverwrite.vi"("overwrite (F)"=TRUE) -> ("overwrite?"=w867:T7)
        n250 = Open/Create/Replace File(file path (use dialog)=w892, error in=w884, operation (0:open)=w867) -> (refnum out=w895:refnum<file>, error out=w894:errorcluster)  [unwired: 3 in, 1 out]
        n251 = call "4155C Write array to file.vi"("Byte Stream File Refnum"=w895, "Header"=string[] ["V stress completed successfully", ""], "error in (no error)"=w894) -> ("dup refnum"=w897:refnum<file>, "error out"=w896:errorcluster)  [unwired: 2 in]
        n252 = Close File(refnum=w897, error in=w896) -> (error out=w890:errorcluster)  [unwired: 1 out]
      }
      frame "stressI" {
        n253 = Number To Decimal String(number=w911) -> (decimal integer string=w948:string)  [unwired: 1 in]
        n254 = Fract/Exp String To Number(string=w945) -> (number=w920:dbl[])  [unwired: 3 in, 1 out]
        n255 = Concatenate Strings(w932, "-stressI-" ("Substring"), w948, w910, ".txt" ("Substring")) -> (w946:string)
        n256 = String To Path(string=w946) -> (path=w936:path)
        n257 = Index Array(array=w920, index=1 ("Index")) -> (element=w916:dbl)
        n258 = Index Array(array=w920, index=0 ("Index")) -> (element=w917:dbl)
        n259 = call "4155C Config I Stress.vi"("VISA session"=w951, "IDG"=w917, "VDG compliance"=w916, "error in (no error)"=w950, "Display on/off"=TRUE) -> ("dup VISA resource name"=w953:refnum<visa-resource-name>, "error out"=w952:errorcluster)
        n260 = Index Array(array=w920, index=2 ("Index")) -> (element=w918:dbl)
        n261 = call "4155C Apply Stress.vi"("error in (no error)"=w952, "Duration"=w918, "Emergency Stop"=w931, "VISA resource name in"=w953) -> ("error out"=w929:errorcluster, "VISA Resource Name out"=w927:refnum<visa-resource-name>)
        n262 = VISA Write(VISA resource name=w927, write buffer=":DISP ON" ("write buffer (\"\")"), error in (no error)=w929) -> (VISA resource name out=w926:refnum<visa-resource-name>, error out=w928:errorcluster)  [unwired: 1 out]
        n263 = call <vilib>:"compatOverwrite.vi"("overwrite (F)"=TRUE) -> ("overwrite?"=w915:T7)
        n264 = Open/Create/Replace File(file path (use dialog)=w936, error in=w928, operation (0:open)=w915) -> (refnum out=w939:refnum<file>, error out=w938:errorcluster)  [unwired: 3 in, 1 out]
        n265 = call "4155C Write array to file.vi"("Byte Stream File Refnum"=w939, "Header"=string[] ["I stress completed successfully", ""], "error in (no error)"=w938) -> ("dup refnum"=w941:refnum<file>, "error out"=w940:errorcluster)  [unwired: 2 in]
        n266 = Close File(refnum=w941, error in=w940) -> (error out=w934:errorcluster)  [unwired: 1 out]
      }
      frame "vsu2pulse" {
        n267 = Number To Decimal String(number=w955) -> (decimal integer string=w990:string)  [unwired: 1 in]
        n268 = Fract/Exp String To Number(string=w987) -> (number=w963:dbl[])  [unwired: 3 in, 1 out]
        n269 = Concatenate Strings(w975, "-vsu2-" ("Substring"), w990, w954, ".txt" ("Substring")) -> (w988:string)
        n270 = String To Path(string=w988) -> (path=w979:path)
        n271 = Index Array(array=w963, index=1 ("Index")) -> (element=w962:dbl)
        n272 = Index Array(array=w963, index=0 ("Index")) -> (element=w960:dbl)
        n273 = call "4155C Config VSU2 Stress.vi"("error in (no error)"=w992, "VSU2"=w960, "Display on/off"=TRUE, "VISA session"=w993) -> ("error out"=w994:errorcluster, "dup VISA resource name"=w995:refnum<visa-resource-name>)
        n274 = call "4155C Apply Stress.vi"("error in (no error)"=w994, "Duration"=w962, "Emergency Stop"=w974, "VISA resource name in"=w995) -> ("error out"=w972:errorcluster, "VISA Resource Name out"=w970:refnum<visa-resource-name>)
        n275 = VISA Write(VISA resource name=w970, write buffer=":DISP ON" ("write buffer (\"\")"), error in (no error)=w972) -> (VISA resource name out=w969:refnum<visa-resource-name>, error out=w971:errorcluster)  [unwired: 1 out]
        n276 = call <vilib>:"compatOverwrite.vi"("overwrite (F)"=TRUE) -> ("overwrite?"=w959:T7)
        n277 = Open/Create/Replace File(file path (use dialog)=w979, error in=w971, operation (0:open)=w959) -> (refnum out=w982:refnum<file>, error out=w981:errorcluster)  [unwired: 3 in, 1 out]
        n278 = call "4155C Write array to file.vi"("Byte Stream File Refnum"=w982, "Header"=string[] ["VSU2 pulse completed successfully", ""], "error in (no error)"=w981) -> ("dup refnum"=w984:refnum<file>, "error out"=w983:errorcluster)  [unwired: 2 in]
        n279 = Close File(refnum=w984, error in=w983) -> (error out=w977:errorcluster)  [unwired: 1 out]
      }
      frame "sample-fpp" {
        w1008 = string[] ["Time /s", "Id VgVd /A", "Ig VgVd /A", "Vp1 VgVd /V", "Vp2 VgVd /V"] ("Header")
        w1012 = "%d" ("format string")
        n280 = Number To Decimal String(number=w997) -> (decimal integer string=w1060:string)  [unwired: 1 in]
        n281 = Fract/Exp String To Number(string=w1057) -> (number=w1045:dbl[])  [unwired: 3 in, 1 out]
        n282 = Concatenate Strings(w1051, "-samplefpp-" ("Substring"), w1060, w996, ".txt" ("Substring")) -> (w1058:string)
        n283 = String To Path(string=w1058) -> (path=w1020:path)
        n284 = Index Array(array=w1045, index=0 ("Index")) -> (element=w1006:dbl)
        n285 = Index Array(array=w1045, index=1 ("Index")) -> (element=w1005:dbl)
        n286 = Index Array(array=w1045, index=2 ("Index")) -> (element=w1053:dbl)
        n287 = Index Array(array=w1045, index=3 ("Index")) -> (element=w1043:dbl)
        n288 = call "4155C Config Sampling Measurements FPP.vi"("VISA session"=w1063, "Num Points"=w1053, "Vg"=w1006, "Display on/off"=TRUE, "Gate Compliance"=w1052, "Drain Compliance"=w1061, "Standby"="Standby", "error in (no error)"=w1062, "Timings"=w1050, "Vd"=w1005, "Sample time"=w1043) -> ("dup VISA resource name"=w1022:refnum<visa-resource-name>, "error out"=w1021:errorcluster)  [unwired: 3 in]
        n289 = Number To Decimal String(number=w1006) -> (decimal integer string=w1032:string)  [unwired: 1 in]
        n290 = call "4155C Take Sample FPP.vi"("VISA resource name in"=w1022, "error in (no error)"=w1021, "Emergency Stop"=w1023) -> ("Time"=w1027:dbl[], "Vp1"=w1037:dbl[], "VISA Resource Name out"=w1003:refnum<visa-resource-name>, "Ig"=w1025:dbl[], "Id"=w1026:dbl[], "Vp2"=w1035:dbl[], "error out"=w1024:errorcluster)  [unwired: 10 in]
        n291 = Insert Into Array(array=dbl[][] [] ("Input Array"), new element=w1027) -> (w1041:dbl[][])  [unwired: 2 in]
        n292 = Number To Decimal String(number=w1005) -> (decimal integer string=w1030:string)  [unwired: 1 in]
        n293 = Insert Into Array(array=w1041, new element=w1026) -> (w1040:dbl[][])  [unwired: 2 in]
        n294 = Concatenate Strings("(Vg = " ("Substring"), w1032, "V, Vd = " ("Substring"), w1030, "V)" ("Substring")) -> (w1028:string)
        n295 = Insert Into Array(array=w1040, new element=w1025) -> (w1039:dbl[][])  [unwired: 2 in]
        n296 = Insert Into Array(array=w1039, new element=w1037) -> (w1036:dbl[][])  [unwired: 2 in]
        n297 = Insert Into Array(array=w1036, new element=w1035) -> (w1004:dbl[][])  [unwired: 2 in]
        n298 = call <vilib>:"compatOverwrite.vi"("overwrite (F)"=TRUE) -> ("overwrite?"=w1001:T7)
        n299 = Open/Create/Replace File(file path (use dialog)=w1020, error in=w1024, operation (0:open)=w1001) -> (refnum out=w1017:refnum<file>, error out=w1018:errorcluster)  [unwired: 3 in, 1 out]
        n300 = Array To Spreadsheet String(array=w1008, 3:w1012) -> (spreadsheet string=w1014:string)  [unwired: 1 in]
        n301 = Transpose 2D Array(2D array=w1004) -> (transposed array=w1034:dbl[][])
        n302 = Search and Replace String(replace all?=TRUE ("replace all? (F)"), input string=w1014, search string="VgVd", replace string=w1028) -> (result string=w1010:string)  [unwired: 4 in, 3 out]
        n303 = Spreadsheet String To Array(format string=w1012, spreadsheet string=w1010, array type (2D Dbl)=w1008) -> (array=w1009:string[])  [unwired: 1 in]
        n304 = call "4155C Write array to file.vi"("Byte Stream File Refnum"=w1017, "Header"=w1009, "Data Array"=w1034, "error in (no error)"=w1018) -> ("dup refnum"=w1015:refnum<file>, "error out"=w1016:errorcluster)  [unwired: 1 in]
        n305 = Close File(refnum=w1015, error in=w1016) -> (error out=w1002:errorcluster)  [unwired: 1 out]
      }
      frame "resample-fpp" {
        w1078 = string[] ["Time /s", "Id VgVd /A", "Ig VgVd /A", "Vp1 VgVd /V", "Vp2 VgVd /V"] ("Header")
        w1082 = "%d" ("format string")
        n306 = Number To Decimal String(number=w1064) -> (decimal integer string=w1122:string)  [unwired: 1 in]
        n307 = Fract/Exp String To Number(string=w1119) -> (number=w1071:dbl[])  [unwired: 3 in, 1 out]
        n308 = Concatenate Strings(w1115, "-resamplefpp-" ("Substring"), w1122, w1065, ".txt" ("Substring")) -> (w1120:string)
        n309 = String To Path(string=w1120) -> (path=w1090:path)
        n310 = Index Array(array=w1071, index=0 ("Index")) -> (element=w1077:dbl)
        n311 = Index Array(array=w1071, index=1 ("Index")) -> (element=w1076:dbl)
        n312 = Number To Decimal String(number=w1077) -> (decimal integer string=w1100:string)  [unwired: 1 in]
        n313 = call "4155C Take Sample FPP.vi"("VISA resource name in"=w1073, "error in (no error)"=w1072, "Emergency Stop"=w1091) -> ("Time"=w1095:dbl[], "Vp1"=w1105:dbl[], "VISA Resource Name out"=w1075:refnum<visa-resource-name>, "Ig"=w1093:dbl[], "Id"=w1094:dbl[], "Vp2"=w1103:dbl[], "error out"=w1092:errorcluster)  [unwired: 10 in]
        n314 = Insert Into Array(array=dbl[][] [] ("Input Array"), new element=w1095) -> (w1109:dbl[][])  [unwired: 2 in]
        n315 = Number To Decimal String(number=w1076) -> (decimal integer string=w1098:string)  [unwired: 1 in]
        n316 = Insert Into Array(array=w1109, new element=w1094) -> (w1108:dbl[][])  [unwired: 2 in]
        n317 = Concatenate Strings("(Vg = " ("Substring"), w1100, "V, Vd = " ("Substring"), w1098, "V)" ("Substring")) -> (w1096:string)
        n318 = Insert Into Array(array=w1108, new element=w1093) -> (w1107:dbl[][])  [unwired: 2 in]
        n319 = Insert Into Array(array=w1107, new element=w1105) -> (w1104:dbl[][])  [unwired: 2 in]
        n320 = Insert Into Array(array=w1104, new element=w1103) -> (w1070:dbl[][])  [unwired: 2 in]
        n321 = call <vilib>:"compatOverwrite.vi"("overwrite (F)"=TRUE) -> ("overwrite?"=w1069:T7)
        n322 = Open/Create/Replace File(file path (use dialog)=w1090, error in=w1092, operation (0:open)=w1069) -> (refnum out=w1087:refnum<file>, error out=w1088:errorcluster)  [unwired: 3 in, 1 out]
        n323 = Array To Spreadsheet String(array=w1078, 3:w1082) -> (spreadsheet string=w1084:string)  [unwired: 1 in]
        n324 = Transpose 2D Array(2D array=w1070) -> (transposed array=w1102:dbl[][])
        n325 = Search and Replace String(replace all?=TRUE ("replace all? (F)"), input string=w1084, search string="VgVd", replace string=w1096) -> (result string=w1080:string)  [unwired: 4 in, 3 out]
        n326 = Spreadsheet String To Array(format string=w1082, spreadsheet string=w1080, array type (2D Dbl)=w1078) -> (array=w1079:string[])  [unwired: 1 in]
        n327 = call "4155C Write array to file.vi"("Byte Stream File Refnum"=w1087, "Header"=w1079, "Data Array"=w1102, "error in (no error)"=w1088) -> ("dup refnum"=w1085:refnum<file>, "error out"=w1086:errorcluster)  [unwired: 1 in]
        n328 = Close File(refnum=w1085, error in=w1086) -> (error out=w1074:errorcluster)  [unwired: 1 out]
      }
      frame "serial" {
        n329 = Index Array(array=w1126, index=0 ("Index")) -> (element=w1125:string)
        n330 = call "Serial write and read v0.4.vi"("Termination char\n(0xA = '\\n' = LF)\n(0xD = '\\r' = CR)"="Termination char\n(0xA = '\\n' = LF)\n(0xD = '\\r' = CR)", "Enable Termination\nChar (T)"="Enable Termination\nChar (T)", "parity"="parity", "stop bits"="stop bits", "string to write"=w1125, "flow control"="flow control", "byte count"="byte count", "Serial Settings:Serial End Mode for Reads"="Serial Settings:Serial End Mode for Reads", "Timeout (ms)"="Timeout (ms)", "error in (no error)"=w1131, "VISA resource name"="VISA resource name", "baud rate"="baud rate", "data bits"="data bits") -> ("read string"=→"Serial port output":string, "error out"=w1130:errorcluster)  [unwired: 1 in]
      }
    }
    n331 = Build Array("Time /s" ("element"), "Id max /A" ("VAR2 Name")) -> (w54:string[])
    n332 = Build Array(w49, w48) -> (w47:dbl[][])
    n333 = Transpose 2D Array(2D array=w47) -> (transposed array=w46:dbl[][])
    n334 = Concatenate Strings(w45, "-Ion-", ".txt" ("Suffix")) -> (w62:string)
    n335 = Array To Spreadsheet String(array=w54, 3:"" ("format string")) -> (spreadsheet string=w53:string)  [unwired: 1 in]
    n336 = Array To Spreadsheet String(array=w46, 3:"%e" ("format string")) -> (spreadsheet string=w52:string)  [unwired: 1 in]
    n337 = String To Path(string=w62) -> (path=w61:path)
    n338 = Build Array(w53, w52) -> (w51:string[])
    n339 = Write to Text File(file (use dialog)=w61, text=w51) -> (refnum out=w63:refnum<file>, error out=w50:errorcluster)  [unwired: 2 in, 1 out]
    n340 = Close File(refnum=w63, error in=w50) -> ()  [unwired: 2 out]
    "Line running" <- w73
    "Total lines" <- w72
  }
  "error out" <- w1
